vi "Main.vi"() -> ()   [LabVIEW 2013]
uses:
  <vilib>/Utility/error.llb/DialogType.ctl
  <vilib>/Utility/miscctls.llb/LVFontTypeDef.ctl
panel:
  out "Buv con ID":refnum<k5>
  out "LoadVolt":bool
  out "LoadPhase":bool
  in  "Tab Control":enum32{"ЛИНЗЫ ПОСТ. ТОКА", "ЛИНЗЫ ИМПУЛЬСНЫЕ"}(tab)
  in  "List of channels":i32(listbox)
  in  "ReadFromFile":bool
  in  "WriteToFile":bool
  out "Дата":string
  out "Время":string
  in  "Comm. current %":dbl=0.5 caption="%" min=0.0 max=100.0 step=0.5
  in  "Common curr. dec":bool
  in  "Common curr. inc":bool
  in  "ConnectAll":bool
  in  "DisconnectAll":bool
  in  "Set Output ON All":bool caption="ВЫХОДЫ ИСТОЧНИКОВ"
  out "текущий ист.":u8
  in  "SetCurrent":dbl min=0.0 max=72.0 step=0.1 format="%#.1g"
  in  "SetVoltage":dbl min=0.0 max=30.0 step=0.1 format="%#.1g"
  in  "SetCurrentB":bool
  in  "SetVoltageB":bool
  in  "SetOutputOffB":bool
  in  "SetOutputOnB":bool
  in  "ConnectChannel":bool
  in  "DisconnectChannel":bool
  in  "SetPhaseEn":bool=TRUE
  in  "BuvPhaseSetB":bool
  in  "SelectedBuvPhase":u16=7000 max=1000 step=1
  out "текущий ист. БУВ":u8
  in  "SelectedBuvOutVolt":dbl min=0.0 max=1000.0 step=0.1 format="%.1f"
  in  "SelectedBuvSetVolB":bool
  in  "Buv Table":i32(listbox)
  in  "Quit":bool=TRUE
  in  "SetCurrentAll":bool
  in  "SetVoltageAll":bool
  in  "Comm. voltage %":dbl caption="%" min=0.0 max=100.0 step=0.5
  in  "Common volt. dec":bool
  in  "Common volt. inc":bool
  in  "№":string="55"
  in  "DeleteChannel":bool
  in  "IP":string="172.16.21.19"
  in  "AddChannel":bool
  out "CURRENTSET":dbl[](array[numeric])
  in  "CurrentModulationOn":bool
  in  "Amp":dbl
  in  "CurrentModulationB":bool
  out "NAME":string[](array[string])
  out "ADRESS":string[](array[string])
  out "VIRef":refnum<vi>[](array[refnum])
  # "ВСЕ ИСТОЧНИКИ"
  # "ИСТОЧНИК №_"
  # "ИСТОЧНИК №_"
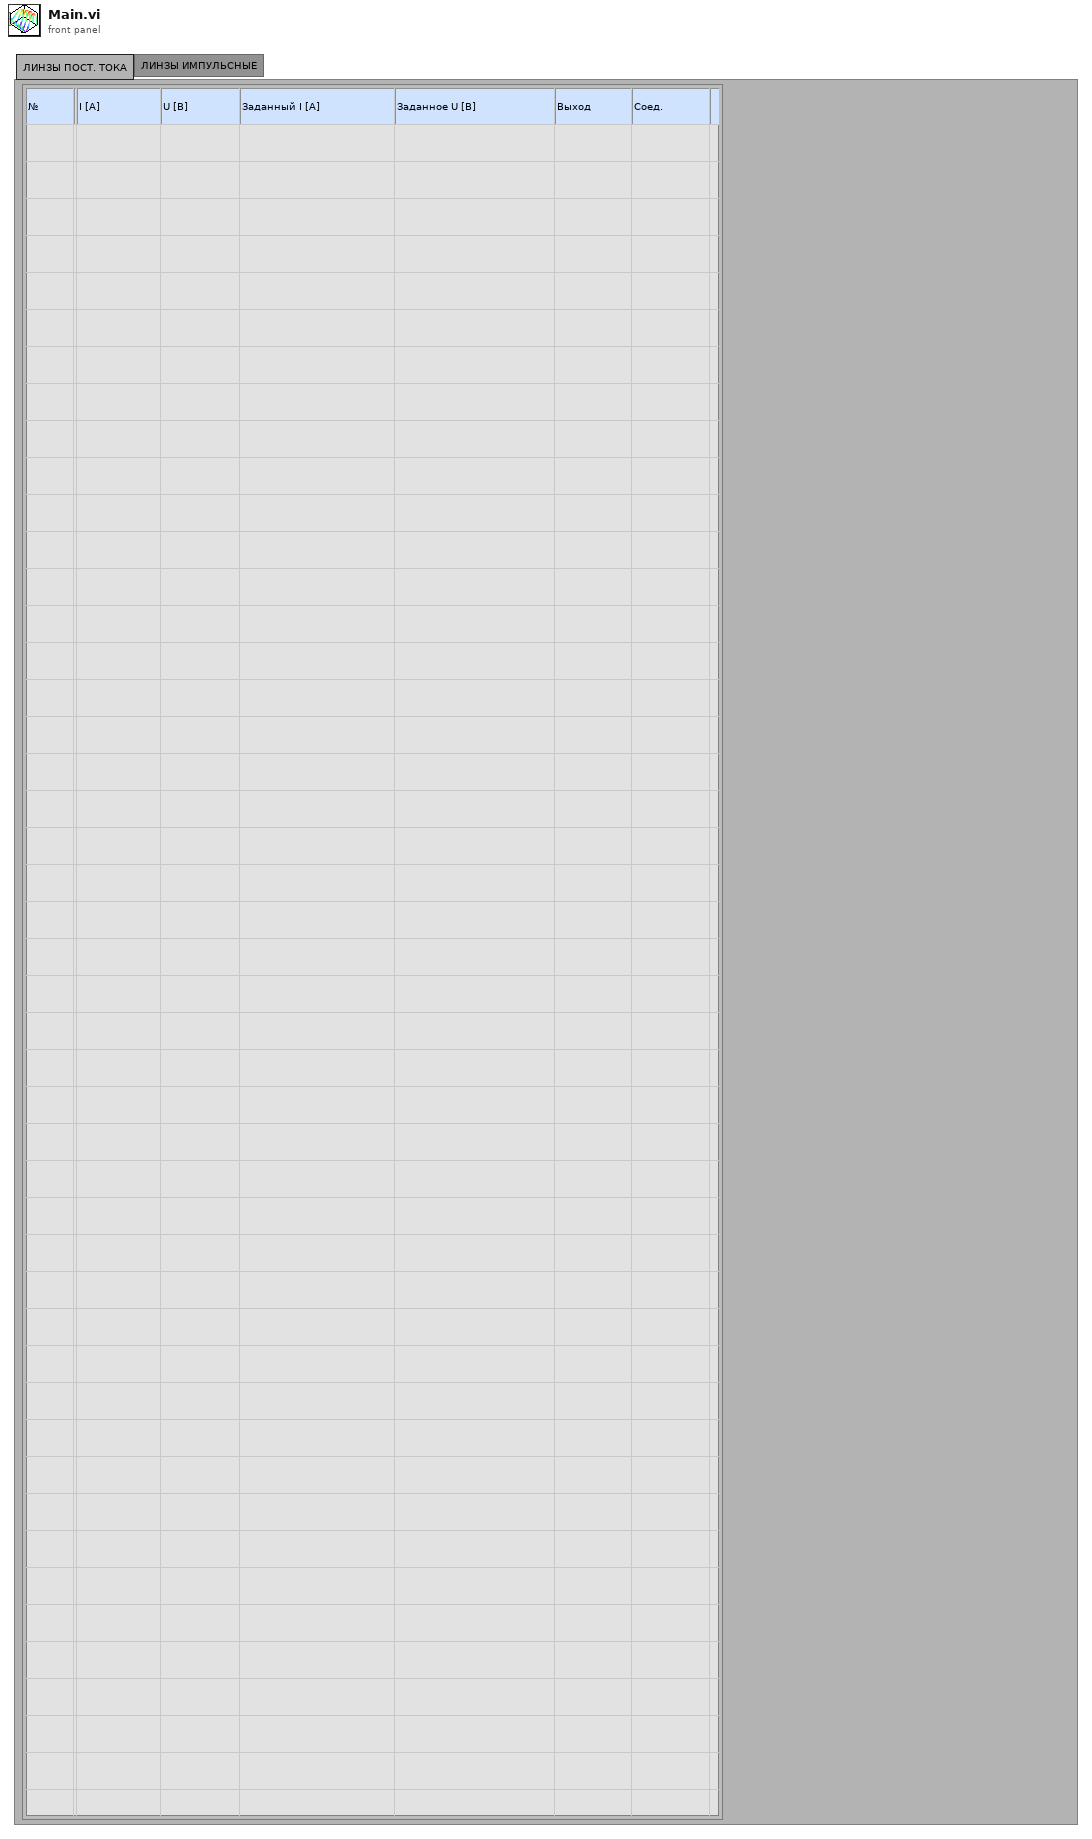
[diagram p1: front panel]
types:
  T1 = enum16{"open", "replace", "create", "open or create", "replace or create", "replace or create with confirmation"}
  T2 = enum8{"Enabled", "Disabled", "Disabled and Grayed Out"}
  T3 = typedef "DialogType.ctl" = u16
  T4 = typedef "LVFontTypeDef.ctl" = cluster{"Font Name":string, "Size":u16, "Bold":bool, "Italic":bool, "Underline":bool, "Strikeout":bool, "Color":u32}
  T5 = enum16{"Standard", "Buffered", "CRLF", "Immediate"}
  T6 = cluster{"milliseconds to wait":i32, "milliseconds to wait":i32}
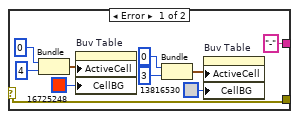
[diagram p6: hidden frame]
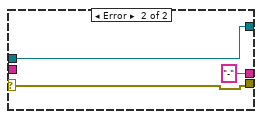
[diagram p7: hidden frame]
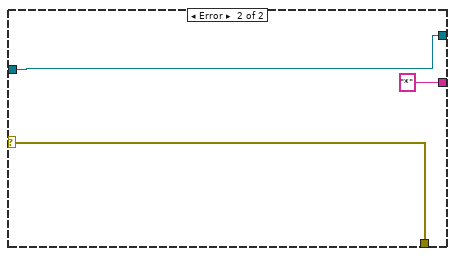
[diagram p8: hidden frame]
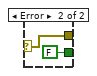
[diagram p10: hidden frame]
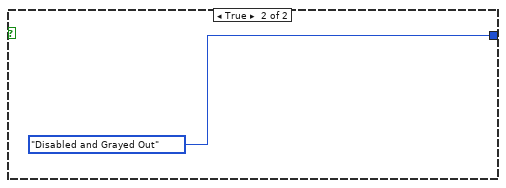
[diagram p11: hidden frame]
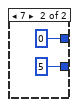
[diagram p13: hidden frame]
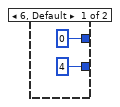
[diagram p14: hidden frame]
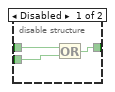
[diagram p15: hidden frame]
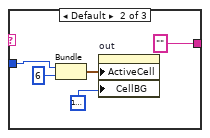
[diagram p16: hidden frame]
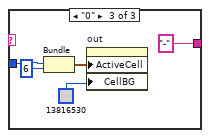
[diagram p17: hidden frame]
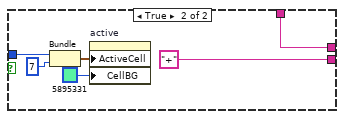
[diagram p18: hidden frame]
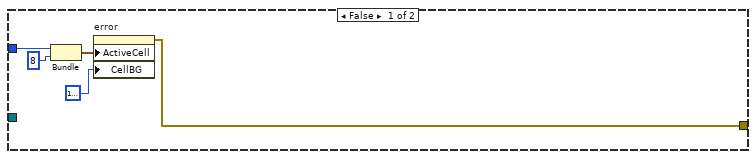
[diagram p19: hidden frame]
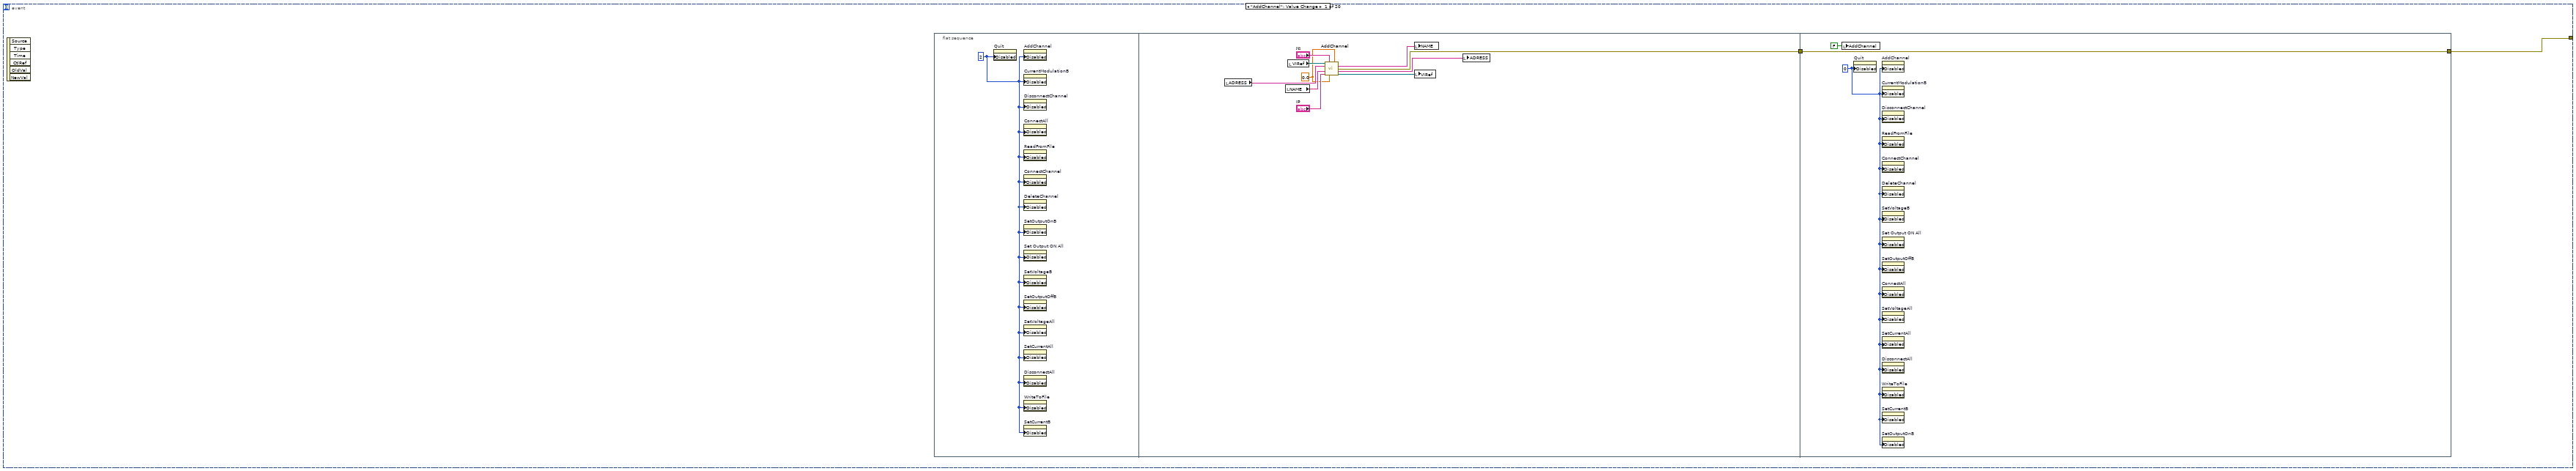
[diagram p20: hidden frame]
diagram:
  w38 = u8 0 ("Disabled")
  w40 = FALSE ("SetOutputOnB")
  w41 = FALSE ("OK Button")
  n1 = event shown="[0] \"Quit\": Value Change" {
    selector: _ -> [_]
    dyn-events: _ -> [_]
    timeout: _ -> [_]
    event "Quit": Value Change {
      n2 = event-data() -> ()  [unwired: 1 in, 1 out]
      n3 = flat-sequence {
        frame #0 {
          w46 = T3 0 items=["no dialog", "OK message", "continue or stop message", "OK message + warnings", "continue/stop + warnings"] ("type of dialog (OK msg:1)")
          n4 = local read "VIRef"() -> (w52:refnum<vi>[])
          n5 = Array Size(array=w52) -> (size(s)=w51:i32)
          n6 = for {
            N: w51 -> [_]
            tunnel: [w53] -> w49 mode=indexing
            i -> [w54]
            n7 = local read "VIRef"() -> (w57:refnum<vi>[])
            n8 = Index Array(array=w57, index=w54) -> (element=w56:refnum<vi>)
            n9 = invoke class="VI" method="Ctrl Val.Set"(reference=w56, "Control Name"="Connect", "Value"=FALSE ("OK Button")) -> (error out=w53:errorcluster)  [unwired: 2 in, 4 out]
          }
          n10 = local read "Buv con ID"() -> (w50:refnum<k5>)
          n11 = TCP Close Connection(connection ID=w50) -> (error out=w48:errorcluster)  [unwired: 2 in, 1 out]
          n12 = Merge Errors(w49, w48) -> (w47:errorcluster)
          n13 = call <vilib>:"General Error Handler.vi"("type of dialog (OK msg:1)"=w46, "error in (no error)"=w47) -> ()  [unwired: 9 in, 5 out]
        }
        frame #1 {
        }
        frame #2 {
          n14 = Stop(stop? (T)=TRUE) -> ()
        }
      }
    }
  }
  n15 = property on="Set Output ON All" class="Bool (strict)"("Disabled"=w38) -> (error out=w30:errorcluster)  [unwired: 2 in, 1 out]
  n16 = property on="SetCurrentAll" class="Bool (strict)"("Disabled"=w38) -> ()  [unwired: 2 in, 2 out]
  n17 = property on="AddChannel" class="Bool (strict)"("Disabled"=w38) -> (error out=w37:errorcluster)  [unwired: 2 in, 1 out]
  n18 = property on="AddChannel" class="Bool (strict)"("Disabled"=u8 0) -> ()  [unwired: 2 in, 2 out]
  n19 = local write "текущий ист."(u8 0 ("текущий ист.")) -> ()
  n20 = property on="IP" class="Str"("Value"="" ("IP")) -> ()  [unwired: 2 in, 2 out]
  n21 = property on="№" class="Str"("Value"="" ("Name")) -> ()  [unwired: 2 in, 2 out]
  n22 = local write "WriteToFile"(w41) -> ()
  n23 = local write "DisconnectChannel"(w41) -> ()
  n24 = local write "ConnectChannel"(w41) -> ()
  n25 = local write "SetCurrentB"(w41) -> ()
  n26 = local write "ReadFromFile"(w41) -> ()
  n27 = local write "AddChannel"(w41) -> ()
  n28 = local write "Quit"(w41) -> ()
  n29 = local write "SetCurrentAll"(w41) -> ()
  n30 = local write "SetVoltageAll"(w41) -> ()
  n31 = local write "DeleteChannel"(w41) -> ()
  n32 = local write "SetVoltageB"(w41) -> ()
  n33 = local write "SetOutputOnB"(w40) -> ()
  n34 = local write "ConnectAll"(w40) -> ()
  n35 = local write "SetOutputOffB"(w40) -> ()
  n36 = local write "DisconnectAll"(w40) -> ()
  n37 = local write "CurrentModulationB"(w40) -> ()
  n38 = local write "CurrentModulationOn"(w40) -> ()
  n39 = for "инициализация цветов и размера ячеек табл." {
    N: 50 -> [_]
    i -> [w62]
    n40 = flat-sequence {
      tunnel: w62 -> [w67]
      tunnel: [w67] -> w61
      tunnel: w61 -> [w106]
      tunnel: [w106] -> w60
      tunnel: w60 -> [w119]
      frame #0 {
        w63 = "Application font" ("Font Name")
        n41 = Bundle(w67, 4) -> (w79:cluster{i32, i32})  [unwired: 1 in]
        n42 = property on="active" class="MCListbox (strict)"("ActiveCell"=w79, "Height"=u32 35 ("Active Cell:Cell Size:Height"), "CellFontSize"=u16 28 ("Size")) -> ()  [unwired: 2 in, 2 out]
        n43 = Bundle(w67, 6) -> (w65:cluster{i32, i32})  [unwired: 1 in]
        n44 = Bundle(w67, 5) -> (w64:cluster{i32, i32})  [unwired: 1 in]
        n45 = Bundle(w67, 0) -> (w90:cluster{i32, i32})  [unwired: 1 in]
        n46 = Bundle(w67, 2) -> (w66:cluster{i32, i32})  [unwired: 1 in]
        n47 = Bundle(w67, 3) -> (w80:cluster{i32, i32})  [unwired: 1 in]
        n48 = Bundle(w67, 1) -> (w89:cluster{i32, i32})  [unwired: 1 in]
        n49 = property on="active" class="MCListbox (strict)"("ActiveCell"=w65, "Height"=u32 35 ("Active Cell:Cell Size:Height"), "CellFontSize"=u16 28 ("Size"), "CellFontName"=w63) -> ()  [unwired: 2 in, 2 out]
        n50 = property on="active" class="MCListbox (strict)"("ActiveCell"=w64, "Height"=u32 35 ("Active Cell:Cell Size:Height"), "CellFontSize"=u16 28 ("Size"), "CellFontName"=w63) -> ()  [unwired: 2 in, 2 out]
        n51 = property on="active" class="MCListbox (strict)"("ActiveCell"=w90, "Height"=u32 35 ("Active Cell:Cell Size:Height"), "CellFontSize"=u16 28 ("Size"), "CellFontName"=w63) -> ()  [unwired: 2 in, 2 out]
        n52 = property on="active" class="MCListbox (strict)"("ActiveCell"=w66, "Height"=u32 35 ("Active Cell:Cell Size:Height"), "CellFontSize"=u16 28 ("Size"), "CellFontName"=w63) -> ()  [unwired: 2 in, 2 out]
        n53 = property on="active" class="MCListbox (strict)"("ActiveCell"=w80, "Height"=u32 35 ("Active Cell:Cell Size:Height"), "CellFontSize"=u16 28 ("Size"), "CellFontName"=w63) -> ()  [unwired: 2 in, 2 out]
        n54 = property on="active" class="MCListbox (strict)"("ActiveCell"=w89, "Height"=u32 35 ("Active Cell:Cell Size:Height"), "CellFontSize"=u16 28 ("Size"), "CellFontName"=w63) -> ()  [unwired: 2 in, 2 out]
      }
      frame #1 {
        w102 = T4 {"Font Name"="Application font", "Size"=28, "Bold"=FALSE, "Italic"=FALSE, "Underline"=FALSE, "Strikeout"=FALSE, "Color"=6908265} ("Active Cell:Cell Font")
        w97 = T4 {"Font Name"="Application font", "Size"=30, "Bold"=TRUE, "Italic"=FALSE, "Underline"=FALSE, "Strikeout"=FALSE, "Color"=2263842} ("Active Cell:Cell Font")
        n55 = Bundle(w106, 4) -> (w99:cluster{i32, i32})  [unwired: 1 in]
        n56 = Bundle(w106, 3) -> (w93:cluster{i32, i32})  [unwired: 1 in]
        n57 = Bundle(w106, 2) -> (w96:cluster{i32, i32})  [unwired: 1 in]
        n58 = Bundle(w106, 0) -> (w104:cluster{i32, i32})  [unwired: 1 in]
        n59 = Bundle(w106, 5) -> (w100:cluster{i32, i32})  [unwired: 1 in]
        n60 = property on="active" class="MCListbox (strict)"("ActiveCell"=w99, "CellFont"=w102) -> ()  [unwired: 2 in, 2 out]
        n61 = property on="active" class="MCListbox (strict)"("ActiveCell"=w93, "CellFont"=w97) -> ()  [unwired: 2 in, 2 out]
        n62 = property on="active" class="MCListbox (strict)"("ActiveCell"=w96, "CellFont"=w97) -> ()  [unwired: 2 in, 2 out]
        n63 = property on="active" class="MCListbox (strict)"("ActiveCell"=w104, "CellFont"=T4 {"Font Name"="Application font", "Size"=28, "Bold"=FALSE, "Italic"=FALSE, "Underline"=FALSE, "Strikeout"=FALSE, "Color"=0} ("Active Cell:Cell Font")) -> ()  [unwired: 2 in, 2 out]
        n64 = property on="active" class="MCListbox (strict)"("ActiveCell"=w100, "CellFont"=w102) -> ()  [unwired: 2 in, 2 out]
      }
      frame #2 {
        w118 = T4 {"Font Name"="Application font", "Size"=28, "Bold"=FALSE, "Italic"=FALSE, "Underline"=FALSE, "Strikeout"=FALSE, "Color"=0} ("Active Cell:Cell Font")
        n65 = Bundle(w119, 6) -> (w113:cluster{i32, i32})  [unwired: 1 in]
        n66 = Bundle(w119, 8) -> (w114:cluster{i32, i32})  [unwired: 1 in]
        n67 = Bundle(w119, 7) -> (w115:cluster{i32, i32})  [unwired: 1 in]
        n68 = property on="active" class="MCListbox (strict)"("ActiveCell"=w113, "CellBG"=u32 16777225) -> (error out=w112:errorcluster)  [unwired: 2 in, 1 out]
        n69 = property on="error" class="MCListbox (strict)"("ActiveCell"=w114, "CellBG"=u32 16777225) -> ()  [unwired: 2 in, 2 out]
        n70 = property on="out" class="MCListbox (strict)"("ActiveCell"=w115, "CellBG"=u32 16777225) -> (error out=w116:errorcluster)  [unwired: 2 in, 1 out]
        n71 = property on="active" class="MCListbox (strict)"(error in=w112, "ActiveCell"=w113, "CellFont"=w118) -> ()  [unwired: 1 in, 2 out]
        n72 = property on="active" class="MCListbox (strict)"(error in=w116, "ActiveCell"=w115, "CellFont"=w118) -> ()  [unwired: 1 in, 2 out]
      }
    }
  }
  n73 = while {
    stop <- FALSE stop-if-true
    n74 = event shown="[13] \"SetOutputOnB\": Value Change" {
      selector: _ -> [_ _ _ _ _ _ _ _ _ _ _ _ _ _ _ _ _ _ _ _]
      dyn-events: _ -> [_ _ _ _ _ _ _ _ _ _ _ _ _ _ _ _ _ _ _ _]
      timeout: _ -> [_ _ _ _ _ _ _ _ _ _ _ _ _ _ _ _ _ _ _ _]
      tunnel: [w123 _ _ _ w227 w243 w259 w303 w347 w362 w388 w404 w420 w437 w458 w481 w499 w550 w624 w647] -> w120
      event "AddChannel": Value Change {
        n75 = event-data() -> ()  [unwired: 7 out]
        n76 = flat-sequence {
          tunnel: [w126] -> w124
          tunnel: [w136] -> w123
          tunnel: w124 -> [w136]
          frame #0 {
            w125 = u8 2 ("Disabled")
            n77 = property on="Quit" class="Bool (strict)"("Disabled"=w125) -> ()  [unwired: 2 in, 2 out]
            n78 = property on="AddChannel" class="Bool (strict)"("Disabled"=w125) -> ()  [unwired: 2 in, 2 out]
            n79 = property on="CurrentModulationB" class="Bool (strict)"("Disabled"=w125) -> ()  [unwired: 2 in, 2 out]
            n80 = property on="DisconnectChannel" class="Bool (strict)"("Disabled"=w125) -> ()  [unwired: 2 in, 2 out]
            n81 = property on="ConnectAll" class="Bool (strict)"("Disabled"=w125) -> ()  [unwired: 2 in, 2 out]
            n82 = property on="ReadFromFile" class="Bool (strict)"("Disabled"=w125) -> ()  [unwired: 2 in, 2 out]
            n83 = property on="ConnectChannel" class="Bool (strict)"("Disabled"=w125) -> ()  [unwired: 2 in, 2 out]
            n84 = property on="DeleteChannel" class="Bool (strict)"("Disabled"=w125) -> ()  [unwired: 2 in, 2 out]
            n85 = property on="SetOutputOnB" class="Bool (strict)"("Disabled"=w125) -> ()  [unwired: 2 in, 2 out]
            n86 = property on="Set Output ON All" class="Bool (strict)"("Disabled"=w125) -> ()  [unwired: 2 in, 2 out]
            n87 = property on="SetVoltageB" class="Bool (strict)"("Disabled"=w125) -> ()  [unwired: 2 in, 2 out]
            n88 = property on="SetOutputOffB" class="Bool (strict)"("Disabled"=w125) -> ()  [unwired: 2 in, 2 out]
            n89 = property on="SetVoltageAll" class="Bool (strict)"("Disabled"=w125) -> ()  [unwired: 2 in, 2 out]
            n90 = property on="SetCurrentAll" class="Bool (strict)"("Disabled"=w125) -> ()  [unwired: 2 in, 2 out]
            n91 = property on="DisconnectAll" class="Bool (strict)"("Disabled"=w125) -> ()  [unwired: 2 in, 2 out]
            n92 = property on="WriteToFile" class="Bool (strict)"("Disabled"=w125) -> ()  [unwired: 2 in, 2 out]
            n93 = property on="SetCurrentB" class="Bool (strict)"("Disabled"=w125) -> ()  [unwired: 2 in, 2 out]
          }
          frame #1 {
            w127 = 0.0 ("SetVoltage")
            n94 = local read "ADRESS"() -> (w133:string[])
            n95 = local read "NAME"() -> (w132:string[])
            n96 = local read "VIRef"() -> (w131:refnum<vi>[])
            n97 = call "AddChannel.vi"("VIRef"=w131, "Name"="№", "SetCurrent"=w127, "ADRESS"=w133, "NAME"=w132, "Address"="IP", "SetVoltage"=w127) -> ("NAMEOut"=w128:string[], "error out"=w126:errorcluster, "ADRESSOut"=w129:string[], "VIRefOut"=w130:refnum<vi>[])  [unwired: 1 in, 4 out]
            n98 = local write "NAME"(w128) -> ()
            n99 = local write "VIRef"(w130) -> ()
            n100 = local write "ADRESS"(w129) -> ()
          }
          frame #2 {
            w137 = u8 0 ("Disabled")
            n101 = local write "AddChannel"(FALSE ("AddChannel")) -> ()
            n102 = property on="Quit" class="Bool (strict)"("Disabled"=w137) -> ()  [unwired: 2 in, 2 out]
            n103 = property on="AddChannel" class="Bool (strict)"("Disabled"=w137) -> ()  [unwired: 2 in, 2 out]
            n104 = property on="CurrentModulationB" class="Bool (strict)"("Disabled"=w137) -> ()  [unwired: 2 in, 2 out]
            n105 = property on="DisconnectChannel" class="Bool (strict)"("Disabled"=w137) -> ()  [unwired: 2 in, 2 out]
            n106 = property on="ReadFromFile" class="Bool (strict)"("Disabled"=w137) -> ()  [unwired: 2 in, 2 out]
            n107 = property on="ConnectChannel" class="Bool (strict)"("Disabled"=w137) -> ()  [unwired: 2 in, 2 out]
            n108 = property on="DeleteChannel" class="Bool (strict)"("Disabled"=w137) -> ()  [unwired: 2 in, 2 out]
            n109 = property on="SetVoltageB" class="Bool (strict)"("Disabled"=w137) -> ()  [unwired: 2 in, 2 out]
            n110 = property on="Set Output ON All" class="Bool (strict)"("Disabled"=w137) -> ()  [unwired: 2 in, 2 out]
            n111 = property on="SetOutputOffB" class="Bool (strict)"("Disabled"=w137) -> ()  [unwired: 2 in, 2 out]
            n112 = property on="ConnectAll" class="Bool (strict)"("Disabled"=w137) -> ()  [unwired: 2 in, 2 out]
            n113 = property on="SetVoltageAll" class="Bool (strict)"("Disabled"=w137) -> ()  [unwired: 2 in, 2 out]
            n114 = property on="SetCurrentAll" class="Bool (strict)"("Disabled"=w137) -> ()  [unwired: 2 in, 2 out]
            n115 = property on="DisconnectAll" class="Bool (strict)"("Disabled"=w137) -> ()  [unwired: 2 in, 2 out]
            n116 = property on="WriteToFile" class="Bool (strict)"("Disabled"=w137) -> ()  [unwired: 2 in, 2 out]
            n117 = property on="SetCurrentB" class="Bool (strict)"("Disabled"=w137) -> ()  [unwired: 2 in, 2 out]
            n118 = property on="SetOutputOnB" class="Bool (strict)"("Disabled"=w137) -> ()  [unwired: 2 in, 2 out]
          }
        }
      }
      event "List of channels": Mouse Down {
        # "Работа с выбранным источником"
        n119 = event-data() -> ()  [unwired: 2 out]
        n120 = property on="List of channels" class="MCListbox (strict)"() -> ("ItemNames"=w142:string[][])  [unwired: 2 in, 2 out]
        n121 = property on="List of channels" class="MCListbox (strict)"() -> ("Value"=w141:i32)  [unwired: 2 in, 2 out]
        n122 = Index Array(array=w142, index (row)=w141) -> (element=w140:string[])  [unwired: 1 in]
        n123 = Empty Array?(array=w140) -> (empty?=w139:bool)
        n124 = case shown="False" w139 {
          tunnel: w140 -> [w143 _]
          frame False {
            n125 = flat-sequence {
              tunnel: w143 -> [w149]
              tunnel: [w149] -> w144
              tunnel: w144 -> [w162]
              frame #0 {
                n126 = Index Array(array=w149, index=0) -> (element=w152:string)
                n127 = Index Array(array=w149, index=7) -> (element=w150:string)
                n128 = case shown="\"-\", Default" w150 {
                  tunnel: [T2."Enabled" ("Disabled") T2."Disabled and Grayed Out" ("Disabled")] -> w145
                  tunnel: [w156 w158] -> w146
                  tunnel: [w156 w158] -> w148
                  tunnel: [w156 w158] -> w147
                  frame "-", Default {
                    w156 = T2."Disabled and Grayed Out" ("Disabled")
                  }
                  frame "+" {
                    w158 = T2."Enabled" ("Disabled")
                    # "соединение с ист."
                  }
                }
                n129 = Scan From String(format string="%f", input string=w152) -> (output 1=→"текущий ист.":u8)  [unwired: 3 in, 3 out]
                n130 = property on="DisconnectAll" class="Bool (strict)"("DisabledEnum"=w146) -> ()  [unwired: 2 in, 2 out]
                n131 = property on="DisconnectChannel" class="Bool (strict)"("DisabledEnum"=w146) -> ()  [unwired: 2 in, 2 out]
                n132 = property on="SetOutputOffB" class="Bool (strict)"("DisabledEnum"=w148) -> ()  [unwired: 2 in, 2 out]
                n133 = property on="SetOutputOnB" class="Bool (strict)"("DisabledEnum"=w147) -> ()  [unwired: 2 in, 2 out]
                n134 = property on="ConnectChannel" class="Bool (strict)"("DisabledEnum"=w145) -> ()  [unwired: 2 in, 2 out]
                n135 = property on="ConnectAll" class="Bool (strict)"("DisabledEnum"=w145) -> ()  [unwired: 2 in, 2 out]
              }
              frame #1 {
                n136 = Index Array(array=w162, index=5) -> (element=w167:string)
                n137 = Index Array(array=w162, index=6) -> (element=w170:string)
                n138 = Index Array(array=w162, index=4) -> (element=w164:string)
                n139 = case shown="\"+\"" w170 {
                  tunnel: [T2."Enabled" ("Disabled") T2."Disabled and Grayed Out" ("Disabled") w177] -> w171
                  tunnel: [T2."Disabled and Grayed Out" ("Disabled") T2."Enabled" ("Disabled") w177] -> w172
                  frame "-", Default {
                  }
                  frame "+" {
                  }
                  frame "?" {
                    w177 = T2."Disabled and Grayed Out" ("Disabled")
                  }
                }
                n140 = Scan From String(format string="%f", input string=w167) -> (output 1=w160:dbl)  [unwired: 3 in, 3 out]
                n141 = Scan From String(format string="%f", input string=w164) -> (output 1=w161:dbl)  [unwired: 3 in, 3 out]
                n142 = local write "SetVoltage"(w160) -> ()
                n143 = local write "SetCurrent"(w161) -> ()
                n144 = property on="SetOutputOffB" class="Bool (strict)"("DisabledEnum"=w172) -> ()  [unwired: 2 in, 2 out]
                n145 = property on="SetOutputOnB" class="Bool (strict)"("DisabledEnum"=w171) -> ()  [unwired: 2 in, 2 out]
              }
            }
          }
          frame True {
          }
        }
      }
      event "Buv Table": Mouse Down {
        # "Работа с выбранным источником БУВ"
        n146 = event-data() -> ()  [unwired: 2 out]
        n147 = property on="Buv Table" class="MCListbox (strict)"() -> ("ItemNames"=w181:string[][])  [unwired: 2 in, 2 out]
        n148 = property on="Buv Table" class="MCListbox (strict)"() -> ("Value"=w180:i32)  [unwired: 2 in, 2 out]
        n149 = Index Array(array=w181, index (row)=w180) -> (element=w179:string[])  [unwired: 1 in]
        n150 = Empty Array?(array=w179) -> (empty?=w178:bool)
        n151 = case shown="False" w178 {
          tunnel: w179 -> [w182 _]
          frame False {
            n152 = flat-sequence {
              tunnel: w182 -> [w185]
              tunnel: [w185] -> w183
              tunnel: w183 -> [w195]
              frame #0 {
                n153 = Index Array(array=w185, index=0) -> (element=w188:string)
                n154 = Index Array(array=w185, index=3) -> (element=w186:string)
                n155 = case shown="\"+\"" w186 {
                  frame "-", Default {
                  }
                  frame "+" {
                    # "соединение с ист."
                  }
                }
                n156 = Scan From String(format string="%f", input string=w188) -> (output 1=→"текущий ист. БУВ":u8)  [unwired: 3 in, 3 out]
              }
              frame #1 {
                n157 = disable-structure shown="Disabled" {
                  disable-tunnel: w195 -> [w197 _]
                  frame Disabled {
                    n158 = Index Array(array=w197, index=1) -> (element=w198:string)
                    n159 = Scan From String(format string="%f", input string=w198) -> ()  [unwired: 4 in, 3 out]
                  }
                  frame Enabled {
                  }
                }
                n160 = Index Array(array=w195, index=2) -> (element=w193:string)
                n161 = Scan From String(format string="%f", input string=w193) -> (output 1=w191:dbl)  [unwired: 3 in, 3 out]
                n162 = local write "SelectedBuvOutVolt"(w191) -> ()
              }
            }
          }
          frame True {
          }
        }
      }
      event Panel Close? {
        n163 = event-data() -> ()  [unwired: 5 out]
        n164 = Two Button Dialog(message="Вы уверены, что хотите закрыть программу?", 1:"Нет" ("F button name (\"Cancel\")"), 2:"Да" ("T button name (\"OK\")")) -> (T button?=w203:bool)
        n165 = case shown="True" w203 {
          frame False {
          }
          frame True {
            n166 = disable-structure shown="Disabled" {
              frame Disabled {
                n167 = local read item#-1() -> (w213)
                n168 = TCP Close Connection(connection ID=w213) -> ()  [unwired: 2 in, 2 out]
              }
              frame Enabled {
              }
            }
            n169 = local read "VIRef"() -> (w205:refnum<vi>[])
            n170 = Array Size(array=w205) -> (size(s)=w204:i32)
            n171 = for {
              N: w204 -> [_]
              tunnel: w205 -> [w223]
              tunnel: [w221] -> w212 mode=indexing
              i -> [w224]
              n172 = Index Array(array=w223, index=w224) -> (element=w222:refnum<vi>)
              n173 = invoke class="VI" method="Ctrl Val.Set"(reference=w222, "Control Name"="Connect", "Value"=FALSE) -> (error out=w221:errorcluster)  [unwired: 2 in, 4 out]
            }
            n174 = flat-sequence {
              tunnel: [w215] -> w211
              tunnel: w212 -> [w215]
              frame #0 {
                n175 = Wait (ms)(milliseconds to wait=u32 1000) -> ()  [unwired: 1 out]
              }
            }
            n176 = local read "VIRef"() -> (w206:refnum<vi>[])
            n177 = Array Size(array=w206) -> (size(s)=w207:i32)
            n178 = for {
              N: w207 -> [_]
              tunnel: w206 -> [w219]
              tunnel: [w217] -> w208 mode=indexing
              tunnel: w211 -> [w216] mode=indexing
              i -> [w220]
              n179 = Index Array(array=w219, index=w220) -> (element=w218:refnum<vi>)
              n180 = invoke class="VI" method="Abort VI"(reference=w218, error in=w216) -> (error out=w217:errorcluster)  [unwired: 1 in, 2 out]
            }
            n181 = Merge Errors(w208) -> (w209:errorcluster)
            n182 = call <vilib>:"General Error Handler.vi"("type of dialog (OK msg:1)"=u32 0 ("milliseconds to wait"), "error in (no error)"=w209) -> ()  [unwired: 9 in, 5 out]
          }
        }
        n183 = event-data() -> ()  [unwired: 2 in, 1 out]
      }
      event "SetVoltageAll": Value Change {
        n184 = event-data() -> ()  [unwired: 7 out]
        n185 = flat-sequence {
          tunnel: [w231] -> w229
          tunnel: [w240] -> w228
          tunnel: w229 -> [w240]
          frame #0 {
            w230 = u8 2 ("Disabled")
            n186 = property on="Quit" class="Bool (strict)"("Disabled"=w230) -> ()  [unwired: 2 in, 2 out]
            n187 = property on="AddChannel" class="Bool (strict)"("Disabled"=w230) -> ()  [unwired: 2 in, 2 out]
            n188 = property on="CurrentModulationB" class="Bool (strict)"("Disabled"=w230) -> ()  [unwired: 2 in, 2 out]
            n189 = property on="DisconnectChannel" class="Bool (strict)"("Disabled"=w230) -> ()  [unwired: 2 in, 2 out]
            n190 = property on="ConnectAll" class="Bool (strict)"("Disabled"=w230) -> ()  [unwired: 2 in, 2 out]
            n191 = property on="ReadFromFile" class="Bool (strict)"("Disabled"=w230) -> ()  [unwired: 2 in, 2 out]
            n192 = property on="ConnectChannel" class="Bool (strict)"("Disabled"=w230) -> ()  [unwired: 2 in, 2 out]
            n193 = property on="DeleteChannel" class="Bool (strict)"("Disabled"=w230) -> ()  [unwired: 2 in, 2 out]
            n194 = property on="SetVoltageB" class="Bool (strict)"("Disabled"=w230) -> ()  [unwired: 2 in, 2 out]
            n195 = property on="Set Output ON All" class="Bool (strict)"("Disabled"=w230) -> ()  [unwired: 2 in, 2 out]
            n196 = property on="SetOutputOffB" class="Bool (strict)"("Disabled"=w230) -> ()  [unwired: 2 in, 2 out]
            n197 = property on="SetVoltageAll" class="Bool (strict)"("Disabled"=w230) -> ()  [unwired: 2 in, 2 out]
            n198 = property on="SetCurrentAll" class="Bool (strict)"("Disabled"=w230) -> ()  [unwired: 2 in, 2 out]
            n199 = property on="DisconnectAll" class="Bool (strict)"("Disabled"=w230) -> ()  [unwired: 2 in, 2 out]
            n200 = property on="WriteToFile" class="Bool (strict)"("Disabled"=w230) -> ()  [unwired: 2 in, 2 out]
            n201 = property on="SetCurrentB" class="Bool (strict)"("Disabled"=w230) -> ()  [unwired: 2 in, 2 out]
            n202 = property on="SetOutputOnB" class="Bool (strict)"("Disabled"=w230) -> ()  [unwired: 2 in, 2 out]
          }
          frame #1 {
            n203 = local read "VIRef"() -> (w233:refnum<vi>[])
            n204 = Array Size(array=w233) -> (size(s)=w232:i32)
            n205 = for {
              N: w232 -> [_]
              tunnel: [w234] -> w231 mode=indexing
              i -> [w236]
              n206 = local read "VIRef"() -> (w239:refnum<vi>[])
              n207 = Index Array(array=w239, index=w236) -> (element=w235:refnum<vi>)
              n208 = invoke class="VI" method="Ctrl Val.Set"(reference=w235, "Control Name"="NeedToSetVoltage", "Value"=TRUE ("ConnectChannel")) -> (error out=w234:errorcluster)  [unwired: 2 in, 4 out]
            }
          }
          frame #2 {
            w241 = u8 0 ("Disabled")
            n209 = local write "SetVoltageAll"(FALSE ("SetVoltageAll")) -> ()
            n210 = property on="Quit" class="Bool (strict)"("Disabled"=w241) -> ()  [unwired: 2 in, 2 out]
            n211 = property on="AddChannel" class="Bool (strict)"("Disabled"=w241) -> ()  [unwired: 2 in, 2 out]
            n212 = property on="CurrentModulationB" class="Bool (strict)"("Disabled"=w241) -> ()  [unwired: 2 in, 2 out]
            n213 = property on="DisconnectChannel" class="Bool (strict)"("Disabled"=w241) -> ()  [unwired: 2 in, 2 out]
            n214 = property on="ReadFromFile" class="Bool (strict)"("Disabled"=w241) -> ()  [unwired: 2 in, 2 out]
            n215 = property on="ConnectChannel" class="Bool (strict)"("Disabled"=w241) -> ()  [unwired: 2 in, 2 out]
            n216 = property on="DeleteChannel" class="Bool (strict)"("Disabled"=w241) -> ()  [unwired: 2 in, 2 out]
            n217 = property on="WriteToFile" class="Bool (strict)"("Disabled"=w241) -> ()  [unwired: 2 in, 2 out]
            n218 = property on="Set Output ON All" class="Bool (strict)"("Disabled"=w241) -> ()  [unwired: 2 in, 2 out]
            n219 = property on="SetCurrentB" class="Bool (strict)"("Disabled"=w241) -> ()  [unwired: 2 in, 2 out]
            n220 = property on="ConnectAll" class="Bool (strict)"("Disabled"=w241) -> ()  [unwired: 2 in, 2 out]
            n221 = property on="SetOutputOnB" class="Bool (strict)"("Disabled"=w241) -> ()  [unwired: 2 in, 2 out]
            n222 = property on="SetVoltageB" class="Bool (strict)"("Disabled"=w241) -> ()  [unwired: 2 in, 2 out]
            n223 = property on="SetOutputOffB" class="Bool (strict)"("Disabled"=w241) -> ()  [unwired: 2 in, 2 out]
            n224 = property on="SetVoltageAll" class="Bool (strict)"("Disabled"=w241) -> ()  [unwired: 2 in, 2 out]
            n225 = property on="SetCurrentAll" class="Bool (strict)"("Disabled"=w241) -> ()  [unwired: 2 in, 2 out]
            n226 = property on="DisconnectAll" class="Bool (strict)"("Disabled"=w241) -> ()  [unwired: 2 in, 2 out]
          }
        }
        n227 = Merge Errors(w228) -> (w227:errorcluster)
      }
      event "SetCurrentAll": Value Change {
        n228 = event-data() -> ()  [unwired: 7 out]
        n229 = flat-sequence {
          tunnel: [w247] -> w245
          tunnel: [w256] -> w244
          tunnel: w245 -> [w256]
          frame #0 {
            w246 = u8 2 ("Disabled")
            n230 = property on="Quit" class="Bool (strict)"("Disabled"=w246) -> ()  [unwired: 2 in, 2 out]
            n231 = property on="AddChannel" class="Bool (strict)"("Disabled"=w246) -> ()  [unwired: 2 in, 2 out]
            n232 = property on="CurrentModulationB" class="Bool (strict)"("Disabled"=w246) -> ()  [unwired: 2 in, 2 out]
            n233 = property on="DisconnectChannel" class="Bool (strict)"("Disabled"=w246) -> ()  [unwired: 2 in, 2 out]
            n234 = property on="ConnectAll" class="Bool (strict)"("Disabled"=w246) -> ()  [unwired: 2 in, 2 out]
            n235 = property on="ReadFromFile" class="Bool (strict)"("Disabled"=w246) -> ()  [unwired: 2 in, 2 out]
            n236 = property on="ConnectChannel" class="Bool (strict)"("Disabled"=w246) -> ()  [unwired: 2 in, 2 out]
            n237 = property on="DeleteChannel" class="Bool (strict)"("Disabled"=w246) -> ()  [unwired: 2 in, 2 out]
            n238 = property on="SetOutputOffB" class="Bool (strict)"("Disabled"=w246) -> ()  [unwired: 2 in, 2 out]
            n239 = property on="Set Output ON All" class="Bool (strict)"("Disabled"=w246) -> ()  [unwired: 2 in, 2 out]
            n240 = property on="SetVoltageAll" class="Bool (strict)"("Disabled"=w246) -> ()  [unwired: 2 in, 2 out]
            n241 = property on="SetCurrentAll" class="Bool (strict)"("Disabled"=w246) -> ()  [unwired: 2 in, 2 out]
            n242 = property on="DisconnectAll" class="Bool (strict)"("Disabled"=w246) -> ()  [unwired: 2 in, 2 out]
            n243 = property on="WriteToFile" class="Bool (strict)"("Disabled"=w246) -> ()  [unwired: 2 in, 2 out]
            n244 = property on="SetCurrentB" class="Bool (strict)"("Disabled"=w246) -> ()  [unwired: 2 in, 2 out]
            n245 = property on="SetOutputOnB" class="Bool (strict)"("Disabled"=w246) -> ()  [unwired: 2 in, 2 out]
            n246 = property on="SetVoltageB" class="Bool (strict)"("Disabled"=w246) -> ()  [unwired: 2 in, 2 out]
          }
          frame #1 {
            n247 = local read "VIRef"() -> (w249:refnum<vi>[])
            n248 = Array Size(array=w249) -> (size(s)=w248:i32)
            n249 = for {
              N: w248 -> [_]
              tunnel: [w250] -> w247 mode=indexing
              i -> [w252]
              n250 = local read "VIRef"() -> (w255:refnum<vi>[])
              n251 = Index Array(array=w255, index=w252) -> (element=w251:refnum<vi>)
              n252 = invoke class="VI" method="Ctrl Val.Set"(reference=w251, "Control Name"="NeedToSetCurrent", "Value"=TRUE ("ConnectChannel")) -> (error out=w250:errorcluster)  [unwired: 2 in, 4 out]
            }
          }
          frame #2 {
            w257 = u8 0 ("Disabled")
            n253 = local write "SetCurrentAll"(FALSE ("SetVoltageAll")) -> ()
            n254 = property on="Quit" class="Bool (strict)"("Disabled"=w257) -> ()  [unwired: 2 in, 2 out]
            n255 = property on="AddChannel" class="Bool (strict)"("Disabled"=w257) -> ()  [unwired: 2 in, 2 out]
            n256 = property on="CurrentModulationB" class="Bool (strict)"("Disabled"=w257) -> ()  [unwired: 2 in, 2 out]
            n257 = property on="DisconnectChannel" class="Bool (strict)"("Disabled"=w257) -> ()  [unwired: 2 in, 2 out]
            n258 = property on="ReadFromFile" class="Bool (strict)"("Disabled"=w257) -> ()  [unwired: 2 in, 2 out]
            n259 = property on="ConnectChannel" class="Bool (strict)"("Disabled"=w257) -> ()  [unwired: 2 in, 2 out]
            n260 = property on="DeleteChannel" class="Bool (strict)"("Disabled"=w257) -> ()  [unwired: 2 in, 2 out]
            n261 = property on="WriteToFile" class="Bool (strict)"("Disabled"=w257) -> ()  [unwired: 2 in, 2 out]
            n262 = property on="Set Output ON All" class="Bool (strict)"("Disabled"=w257) -> ()  [unwired: 2 in, 2 out]
            n263 = property on="SetCurrentB" class="Bool (strict)"("Disabled"=w257) -> ()  [unwired: 2 in, 2 out]
            n264 = property on="ConnectAll" class="Bool (strict)"("Disabled"=w257) -> ()  [unwired: 2 in, 2 out]
            n265 = property on="SetOutputOnB" class="Bool (strict)"("Disabled"=w257) -> ()  [unwired: 2 in, 2 out]
            n266 = property on="SetVoltageB" class="Bool (strict)"("Disabled"=w257) -> ()  [unwired: 2 in, 2 out]
            n267 = property on="SetOutputOffB" class="Bool (strict)"("Disabled"=w257) -> ()  [unwired: 2 in, 2 out]
            n268 = property on="SetVoltageAll" class="Bool (strict)"("Disabled"=w257) -> ()  [unwired: 2 in, 2 out]
            n269 = property on="SetCurrentAll" class="Bool (strict)"("Disabled"=w257) -> ()  [unwired: 2 in, 2 out]
            n270 = property on="DisconnectAll" class="Bool (strict)"("Disabled"=w257) -> ()  [unwired: 2 in, 2 out]
          }
        }
        n271 = Merge Errors(w244) -> (w243:errorcluster)
      }
      event "Common curr. inc", "Common curr. dec": Value Change {
        # "Общее управление токами"
        n272 = event-data() -> ()  [unwired: 2 out]
        n273 = local read "ADRESS"() -> (w262:string[])
        n274 = Array Size(array=w262) -> (size(s)=w263:i32)
        n275 = for {
          N: w263 -> [_]
          tunnel: [w272] -> w261 mode=indexing
          i -> [w290]
          n276 = local read "VIRef"() -> (w293:refnum<vi>[])
          n277 = Index Array(array=w293, index=w290) -> (element=w280:refnum<vi>)
          n278 = invoke class="VI" method="Ctrl Val.Get"(reference=w280, "Control Name"="SetCurrentStr") -> (reference out=w274:refnum<vi>, error out=w288:errorcluster, "Get Control Value Variant"=w292:variant)  [unwired: 2 in, 1 out]
          n279 = Variant To Data(error in=w288, type="" ("Control Name"), Variant=w292) -> (data=w287:string, error out=w286:errorcluster)
          n280 = Scan From String(format string="%f", input string=w287, error in=w286) -> (error out=w273:errorcluster, output 1=w271:dbl)  [unwired: 2 in, 2 out]
          n281 = Multiply(x=w271, y="Comm. current %") -> (x*y=w282:dbl)
          n282 = Divide(x=w282, y=100.0) -> (x/y=w284:dbl)
          n283 = local read "Common curr. inc"() -> (w270:bool)
          n284 = local read "Common curr. dec"() -> (w268:bool)
          n285 = case shown="True" w270 {
            tunnel: w284 -> [w298 w302]
            tunnel: w271 -> [w299 w301]
            tunnel: [w299 w300] -> w269
            tunnel: [w298 _] -> w267
            frame False {
            }
            frame True {
              n286 = Add(x=w301, y=w302) -> (x+y=w300:dbl)
            }
          }
          n287 = case shown="False" w268 {
            tunnel: w269 -> [w294 w297]
            tunnel: [w294 w296] -> w266
            tunnel: w267 -> [_ w295]
            frame False {
            }
            frame True {
              n288 = Subtract(x=w297, y=w295) -> (x-y=w296:dbl)
            }
          }
          n289 = invoke class="VI" method="Ctrl Val.Set"(reference=w274, error in=w273, "Control Name"="SetCurrent", "Value"=w266) -> (reference out=w276:refnum<vi>, error out=w275:errorcluster)  [unwired: 1 in, 3 out]
          n290 = invoke class="VI" method="Ctrl Val.Set"(reference=w276, error in=w275, "Control Name"="NeedToSetCurrent", "Value"=TRUE ("ConnectChannel")) -> (error out=w272:errorcluster)  [unwired: 1 in, 4 out]
        }
        n291 = Merge Errors(w261) -> (w260:errorcluster)
        n292 = flat-sequence {
          tunnel: w260 -> [w265]
          tunnel: [w265] -> w259
          frame #0 {
            w264 = FALSE ("ConnectChannel")
            n293 = local write "Common curr. inc"(w264) -> ()
            n294 = local write "Common curr. dec"(w264) -> ()
          }
        }
      }
      event "Common volt. inc", "Common volt. dec": Value Change {
        # "Общее управление напряжением"
        n295 = event-data() -> ()  [unwired: 2 out]
        n296 = local read "ADRESS"() -> (w306:string[])
        n297 = Array Size(array=w306) -> (size(s)=w307:i32)
        n298 = for {
          N: w307 -> [_]
          tunnel: [w317] -> w305 mode=indexing
          i -> [w334]
          n299 = local read "VIRef"() -> (w337:refnum<vi>[])
          n300 = Index Array(array=w337, index=w334) -> (element=w325:refnum<vi>)
          n301 = invoke class="VI" method="Ctrl Val.Get"(reference=w325, "Control Name"="SetVoltageStr") -> (reference out=w319:refnum<vi>, error out=w332:errorcluster, "Get Control Value Variant"=w336:variant)  [unwired: 2 in, 1 out]
          n302 = Variant To Data(error in=w332, type="" ("Control Name"), Variant=w336) -> (data=w331:string, error out=w330:errorcluster)
          n303 = Scan From String(format string="%f", input string=w331, error in=w330) -> (error out=w318:errorcluster, output 1=w316:dbl)  [unwired: 2 in, 2 out]
          n304 = Multiply(x=w316, y="Comm. voltage %") -> (x*y=w326:dbl)
          n305 = Divide(x=w326, y=100.0) -> (x/y=w328:dbl)
          n306 = local read "Common volt. inc"() -> (w315:bool)
          n307 = local read "Common volt. dec"() -> (w313:bool)
          n308 = case shown="True" w315 {
            tunnel: w328 -> [w342 w346]
            tunnel: w316 -> [w343 w345]
            tunnel: [w343 w344] -> w314
            tunnel: [w342 _] -> w312
            frame False {
            }
            frame True {
              n309 = Add(x=w345, y=w346) -> (x+y=w344:dbl)
            }
          }
          n310 = case shown="False" w313 {
            tunnel: w314 -> [w338 w341]
            tunnel: [w338 w340] -> w311
            tunnel: w312 -> [_ w339]
            frame False {
            }
            frame True {
              n311 = Subtract(x=w341, y=w339) -> (x-y=w340:dbl)
            }
          }
          n312 = invoke class="VI" method="Ctrl Val.Set"(reference=w319, error in=w318, "Control Name"="SetVoltage", "Value"=w311) -> (reference out=w321:refnum<vi>, error out=w320:errorcluster)  [unwired: 1 in, 3 out]
          n313 = invoke class="VI" method="Ctrl Val.Set"(reference=w321, error in=w320, "Control Name"="NeedToSetVoltage", "Value"=TRUE ("ConnectChannel")) -> (error out=w317:errorcluster)  [unwired: 1 in, 4 out]
        }
        n314 = Merge Errors(w305) -> (w304:errorcluster)
        n315 = flat-sequence {
          tunnel: w304 -> [w309]
          tunnel: [w309] -> w303
          frame #0 {
            w308 = FALSE ("ConnectChannel")
            n316 = local write "Common volt. inc"(w308) -> ()
            n317 = local write "Common volt. dec"(w308) -> ()
          }
        }
      }
      event "DisconnectChannel": Value Change {
        n318 = event-data() -> ()  [unwired: 7 out]
        n319 = property on="List of channels" class="MCListbox (strict)"() -> ("Value"=w351:i32)  [unwired: 2 in, 2 out]
        n320 = flat-sequence {
          tunnel: w351 -> [w353]
          tunnel: [w353] -> w350
          tunnel: w350 -> [w355]
          tunnel: [w354] -> w348
          tunnel: [w360] -> w349
          tunnel: w348 -> [w360]
          frame #0 {
            w352 = u8 2 ("Disabled")
            n321 = property on="AddChannel" class="Bool (strict)"("Disabled"=w352) -> ()  [unwired: 2 in, 2 out]
            n322 = property on="Set Output ON All" class="Bool (strict)"("Disabled"=w352) -> ()  [unwired: 2 in, 2 out]
            n323 = property on="CurrentModulationB" class="Bool (strict)"("Disabled"=w352) -> ()  [unwired: 2 in, 2 out]
            n324 = property on="ConnectAll" class="Bool (strict)"("Disabled"=w352) -> ()  [unwired: 2 in, 2 out]
            n325 = property on="DisconnectChannel" class="Bool (strict)"("Disabled"=w352) -> ()  [unwired: 2 in, 2 out]
            n326 = property on="ReadFromFile" class="Bool (strict)"("Disabled"=w352) -> ()  [unwired: 2 in, 2 out]
            n327 = property on="Quit" class="Bool (strict)"("Disabled"=w352) -> ()  [unwired: 2 in, 2 out]
            n328 = property on="ConnectChannel" class="Bool (strict)"("Disabled"=w352) -> ()  [unwired: 2 in, 2 out]
            n329 = property on="DeleteChannel" class="Bool (strict)"("Disabled"=w352) -> ()  [unwired: 2 in, 2 out]
            n330 = property on="WriteToFile" class="Bool (strict)"("Disabled"=w352) -> ()  [unwired: 2 in, 2 out]
            n331 = property on="SetCurrentB" class="Bool (strict)"("Disabled"=w352) -> ()  [unwired: 2 in, 2 out]
            n332 = property on="SetOutputOnB" class="Bool (strict)"("Disabled"=w352) -> ()  [unwired: 2 in, 2 out]
            n333 = property on="SetVoltageB" class="Bool (strict)"("Disabled"=w352) -> ()  [unwired: 2 in, 2 out]
            n334 = property on="SetOutputOffB" class="Bool (strict)"("Disabled"=w352) -> ()  [unwired: 2 in, 2 out]
            n335 = property on="SetVoltageAll" class="Bool (strict)"("Disabled"=w352) -> ()  [unwired: 2 in, 2 out]
            n336 = property on="SetCurrentAll" class="Bool (strict)"("Disabled"=w352) -> ()  [unwired: 2 in, 2 out]
            n337 = property on="DisconnectAll" class="Bool (strict)"("Disabled"=w352) -> ()  [unwired: 2 in, 2 out]
          }
          frame #1 {
            w356 = FALSE ("OK Button")
            n338 = local write "DisconnectChannel"(w356) -> ()
            n339 = local read "VIRef"() -> (w358:refnum<vi>[])
            n340 = Index Array(array=w358, index=w355) -> (element=w357:refnum<vi>)
            n341 = invoke class="VI" method="Ctrl Val.Set"(reference=w357, "Control Name"="Connect", "Value"=w356) -> (error out=w354:errorcluster)  [unwired: 2 in, 4 out]
          }
          frame #2 {
            w361 = u8 0 ("Disabled")
            n342 = property on="AddChannel" class="Bool (strict)"("Disabled"=w361) -> ()  [unwired: 2 in, 2 out]
            n343 = property on="CurrentModulationB" class="Bool (strict)"("Disabled"=w361) -> ()  [unwired: 2 in, 2 out]
            n344 = property on="DisconnectChannel" class="Bool (strict)"("Disabled"=w361) -> ()  [unwired: 2 in, 2 out]
            n345 = property on="ConnectAll" class="Bool (strict)"("Disabled"=w361) -> ()  [unwired: 2 in, 2 out]
            n346 = property on="ReadFromFile" class="Bool (strict)"("Disabled"=w361) -> ()  [unwired: 2 in, 2 out]
            n347 = property on="ConnectChannel" class="Bool (strict)"("Disabled"=w361) -> ()  [unwired: 2 in, 2 out]
            n348 = property on="Quit" class="Bool (strict)"("Disabled"=w361) -> ()  [unwired: 2 in, 2 out]
            n349 = property on="DeleteChannel" class="Bool (strict)"("Disabled"=w361) -> ()  [unwired: 2 in, 2 out]
            n350 = property on="SetOutputOffB" class="Bool (strict)"("Disabled"=w361) -> ()  [unwired: 2 in, 2 out]
            n351 = property on="Set Output ON All" class="Bool (strict)"("Disabled"=w361) -> ()  [unwired: 2 in, 2 out]
            n352 = property on="SetVoltageAll" class="Bool (strict)"("Disabled"=w361) -> ()  [unwired: 2 in, 2 out]
            n353 = property on="SetCurrentAll" class="Bool (strict)"("Disabled"=w361) -> ()  [unwired: 2 in, 2 out]
            n354 = property on="DisconnectAll" class="Bool (strict)"("Disabled"=w361) -> ()  [unwired: 2 in, 2 out]
            n355 = property on="WriteToFile" class="Bool (strict)"("Disabled"=w361) -> ()  [unwired: 2 in, 2 out]
            n356 = property on="SetCurrentB" class="Bool (strict)"("Disabled"=w361) -> ()  [unwired: 2 in, 2 out]
            n357 = property on="SetOutputOnB" class="Bool (strict)"("Disabled"=w361) -> ()  [unwired: 2 in, 2 out]
            n358 = property on="SetVoltageB" class="Bool (strict)"("Disabled"=w361) -> ()  [unwired: 2 in, 2 out]
          }
        }
        n359 = Merge Errors(w349) -> (w347:errorcluster)
      }
      event "ConnectChannel": Value Change {
        n360 = event-data() -> ()  [unwired: 7 out]
        n361 = property on="List of channels" class="MCListbox (strict)"() -> ("Value"=w366:i32)  [unwired: 2 in, 2 out]
        n362 = flat-sequence {
          tunnel: w366 -> [w368]
          tunnel: [w368] -> w365
          tunnel: w365 -> [w373]
          tunnel: [w372] -> w363
          tunnel: [w385] -> w364
          tunnel: w363 -> [w385]
          frame #0 {
            w367 = u8 2 ("Disabled")
            n363 = property on="AddChannel" class="Bool (strict)"("Disabled"=w367) -> ()  [unwired: 2 in, 2 out]
            n364 = property on="Set Output ON All" class="Bool (strict)"("Disabled"=w367) -> ()  [unwired: 2 in, 2 out]
            n365 = property on="CurrentModulationB" class="Bool (strict)"("Disabled"=w367) -> ()  [unwired: 2 in, 2 out]
            n366 = property on="ConnectAll" class="Bool (strict)"("Disabled"=w367) -> ()  [unwired: 2 in, 2 out]
            n367 = property on="DisconnectChannel" class="Bool (strict)"("Disabled"=w367) -> ()  [unwired: 2 in, 2 out]
            n368 = property on="ReadFromFile" class="Bool (strict)"("Disabled"=w367) -> ()  [unwired: 2 in, 2 out]
            n369 = property on="Quit" class="Bool (strict)"("Disabled"=w367) -> ()  [unwired: 2 in, 2 out]
            n370 = property on="ConnectChannel" class="Bool (strict)"("Disabled"=w367) -> ()  [unwired: 2 in, 2 out]
            n371 = property on="DeleteChannel" class="Bool (strict)"("Disabled"=w367) -> ()  [unwired: 2 in, 2 out]
            n372 = property on="WriteToFile" class="Bool (strict)"("Disabled"=w367) -> ()  [unwired: 2 in, 2 out]
            n373 = property on="SetCurrentB" class="Bool (strict)"("Disabled"=w367) -> ()  [unwired: 2 in, 2 out]
            n374 = property on="SetOutputOnB" class="Bool (strict)"("Disabled"=w367) -> ()  [unwired: 2 in, 2 out]
            n375 = property on="SetVoltageB" class="Bool (strict)"("Disabled"=w367) -> ()  [unwired: 2 in, 2 out]
            n376 = property on="SetOutputOffB" class="Bool (strict)"("Disabled"=w367) -> ()  [unwired: 2 in, 2 out]
            n377 = property on="SetVoltageAll" class="Bool (strict)"("Disabled"=w367) -> ()  [unwired: 2 in, 2 out]
            n378 = property on="SetCurrentAll" class="Bool (strict)"("Disabled"=w367) -> ()  [unwired: 2 in, 2 out]
            n379 = property on="DisconnectAll" class="Bool (strict)"("Disabled"=w367) -> ()  [unwired: 2 in, 2 out]
          }
          frame #1 {
            n380 = local read "VIRef"() -> (w374:refnum<vi>[])
            n381 = Index Array(array=w374, index=w373) -> (element=w371:refnum<vi>)
            n382 = flat-sequence {
              tunnel: w371 -> [w376]
              tunnel: [w375] -> w369
              tunnel: [w379] -> w370
              tunnel: w369 -> [w379]
              tunnel: [w381] -> w372
              tunnel: w370 -> [w382]
              frame #0 {
                n383 = invoke class="VI" method="Ctrl Val.Set"(reference=w376, "Control Name"="Connect", "Value"=FALSE ("OK Button")) -> (reference out=w375:refnum<vi>)  [unwired: 2 in, 4 out]
              }
              frame #1 {
                n384 = Wait (ms)(milliseconds to wait=u32 1000) -> ()  [unwired: 1 out]
              }
              frame #2 {
                n385 = invoke class="VI" method="Ctrl Val.Set"(reference=w382, "Control Name"="Connect", "Value"=TRUE ("OK Button")) -> (error out=w381:errorcluster)  [unwired: 2 in, 4 out]
              }
            }
          }
          frame #2 {
            w386 = u8 0 ("Disabled")
            n386 = local write "ConnectChannel"(FALSE ("ConnectChannel")) -> ()
            n387 = property on="ConnectAll" class="Bool (strict)"("Disabled"=w386) -> ()  [unwired: 2 in, 2 out]
            n388 = property on="Set Output ON All" class="Bool (strict)"("Disabled"=w386) -> ()  [unwired: 2 in, 2 out]
            n389 = property on="AddChannel" class="Bool (strict)"("Disabled"=w386) -> ()  [unwired: 2 in, 2 out]
            n390 = property on="DisconnectChannel" class="Bool (strict)"("Disabled"=w386) -> ()  [unwired: 2 in, 2 out]
            n391 = property on="ReadFromFile" class="Bool (strict)"("Disabled"=w386) -> ()  [unwired: 2 in, 2 out]
            n392 = property on="ConnectChannel" class="Bool (strict)"("Disabled"=w386) -> ()  [unwired: 2 in, 2 out]
            n393 = property on="Quit" class="Bool (strict)"("Disabled"=w386) -> ()  [unwired: 2 in, 2 out]
            n394 = property on="DeleteChannel" class="Bool (strict)"("Disabled"=w386) -> ()  [unwired: 2 in, 2 out]
            n395 = property on="WriteToFile" class="Bool (strict)"("Disabled"=w386) -> ()  [unwired: 2 in, 2 out]
            n396 = property on="CurrentModulationB" class="Bool (strict)"("Disabled"=w386) -> ()  [unwired: 2 in, 2 out]
            n397 = property on="SetCurrentB" class="Bool (strict)"("Disabled"=w386) -> ()  [unwired: 2 in, 2 out]
            n398 = property on="SetOutputOnB" class="Bool (strict)"("Disabled"=w386) -> ()  [unwired: 2 in, 2 out]
            n399 = property on="SetVoltageB" class="Bool (strict)"("Disabled"=w386) -> ()  [unwired: 2 in, 2 out]
            n400 = property on="SetOutputOffB" class="Bool (strict)"("Disabled"=w386) -> ()  [unwired: 2 in, 2 out]
            n401 = property on="SetVoltageAll" class="Bool (strict)"("Disabled"=w386) -> ()  [unwired: 2 in, 2 out]
            n402 = property on="SetCurrentAll" class="Bool (strict)"("Disabled"=w386) -> ()  [unwired: 2 in, 2 out]
            n403 = property on="DisconnectAll" class="Bool (strict)"("Disabled"=w386) -> ()  [unwired: 2 in, 2 out]
          }
        }
        n404 = Merge Errors(w364) -> (w362:errorcluster)
      }
      event "ConnectAll": Value Change {
        n405 = event-data() -> ()  [unwired: 7 out]
        n406 = flat-sequence {
          tunnel: [w392] -> w389
          tunnel: [w401] -> w390
          tunnel: w389 -> [w401]
          frame #0 {
            w391 = u8 2 ("Disabled")
            n407 = property on="Quit" class="Bool (strict)"("Disabled"=w391) -> ()  [unwired: 2 in, 2 out]
            n408 = property on="ReadFromFile" class="Bool (strict)"("Disabled"=w391) -> ()  [unwired: 2 in, 2 out]
            n409 = property on="CurrentModulationB" class="Bool (strict)"("Disabled"=w391) -> ()  [unwired: 2 in, 2 out]
            n410 = property on="WriteToFile" class="Bool (strict)"("Disabled"=w391) -> ()  [unwired: 2 in, 2 out]
            n411 = property on="ConnectAll" class="Bool (strict)"("Disabled"=w391) -> ()  [unwired: 2 in, 2 out]
            n412 = property on="Set Output ON All" class="Bool (strict)"("Disabled"=w391) -> ()  [unwired: 2 in, 2 out]
            n413 = property on="SetOutputOffB" class="Bool (strict)"("Disabled"=w391) -> ()  [unwired: 2 in, 2 out]
            n414 = property on="AddChannel" class="Bool (strict)"("Disabled"=w391) -> ()  [unwired: 2 in, 2 out]
            n415 = property on="DisconnectChannel" class="Bool (strict)"("Disabled"=w391) -> ()  [unwired: 2 in, 2 out]
            n416 = property on="SetCurrentAll" class="Bool (strict)"("Disabled"=w391) -> ()  [unwired: 2 in, 2 out]
            n417 = property on="SetOutputOnB" class="Bool (strict)"("Disabled"=w391) -> ()  [unwired: 2 in, 2 out]
            n418 = property on="ConnectChannel" class="Bool (strict)"("Disabled"=w391) -> ()  [unwired: 2 in, 2 out]
            n419 = property on="DeleteChannel" class="Bool (strict)"("Disabled"=w391) -> ()  [unwired: 2 in, 2 out]
            n420 = property on="SetCurrentB" class="Bool (strict)"("Disabled"=w391) -> ()  [unwired: 2 in, 2 out]
            n421 = property on="SetVoltageB" class="Bool (strict)"("Disabled"=w391) -> ()  [unwired: 2 in, 2 out]
            n422 = property on="SetVoltageAll" class="Bool (strict)"("Disabled"=w391) -> ()  [unwired: 2 in, 2 out]
            n423 = property on="DisconnectAll" class="Bool (strict)"("Disabled"=w391) -> ()  [unwired: 2 in, 2 out]
          }
          frame #1 {
            n424 = local read "VIRef"() -> (w394:refnum<vi>[])
            n425 = Array Size(array=w394) -> (size(s)=w393:i32)
            n426 = for {
              N: w393 -> [_]
              tunnel: [w395] -> w392 mode=indexing
              i -> [w396]
              n427 = local read "VIRef"() -> (w399:refnum<vi>[])
              n428 = Index Array(array=w399, index=w396) -> (element=w398:refnum<vi>)
              n429 = invoke class="VI" method="Ctrl Val.Set"(reference=w398, "Control Name"="Connect", "Value"=TRUE ("OK Button")) -> (error out=w395:errorcluster)  [unwired: 2 in, 4 out]
            }
          }
          frame #2 {
            w402 = u8 0 ("Disabled")
            n430 = local write "ConnectAll"(FALSE ("ConnectChannel")) -> ()
            n431 = property on="Quit" class="Bool (strict)"("Disabled"=w402) -> ()  [unwired: 2 in, 2 out]
            n432 = property on="AddChannel" class="Bool (strict)"("Disabled"=w402) -> ()  [unwired: 2 in, 2 out]
            n433 = property on="DisconnectChannel" class="Bool (strict)"("Disabled"=w402) -> ()  [unwired: 2 in, 2 out]
            n434 = property on="ConnectAll" class="Bool (strict)"("Disabled"=w402) -> ()  [unwired: 2 in, 2 out]
            n435 = property on="Set Output ON All" class="Bool (strict)"("Disabled"=w402) -> ()  [unwired: 2 in, 2 out]
            n436 = property on="SetOutputOffB" class="Bool (strict)"("Disabled"=w402) -> ()  [unwired: 2 in, 2 out]
            n437 = property on="SetCurrentAll" class="Bool (strict)"("Disabled"=w402) -> ()  [unwired: 2 in, 2 out]
            n438 = property on="ConnectChannel" class="Bool (strict)"("Disabled"=w402) -> ()  [unwired: 2 in, 2 out]
            n439 = property on="SetVoltageAll" class="Bool (strict)"("Disabled"=w402) -> ()  [unwired: 2 in, 2 out]
            n440 = property on="SetOutputOnB" class="Bool (strict)"("Disabled"=w402) -> ()  [unwired: 2 in, 2 out]
            n441 = property on="CurrentModulationB" class="Bool (strict)"("Disabled"=w402) -> ()  [unwired: 2 in, 2 out]
            n442 = property on="DisconnectAll" class="Bool (strict)"("Disabled"=w402) -> ()  [unwired: 2 in, 2 out]
            n443 = property on="ReadFromFile" class="Bool (strict)"("Disabled"=w402) -> ()  [unwired: 2 in, 2 out]
            n444 = property on="WriteToFile" class="Bool (strict)"("Disabled"=w402) -> ()  [unwired: 2 in, 2 out]
            n445 = property on="SetCurrentB" class="Bool (strict)"("Disabled"=w402) -> ()  [unwired: 2 in, 2 out]
            n446 = property on="SetVoltageB" class="Bool (strict)"("Disabled"=w402) -> ()  [unwired: 2 in, 2 out]
            n447 = property on="DeleteChannel" class="Bool (strict)"("Disabled"=w402) -> ()  [unwired: 2 in, 2 out]
          }
        }
        n448 = Merge Errors(w390) -> (w388:errorcluster)
      }
      event "DisconnectAll": Value Change {
        n449 = event-data() -> ()  [unwired: 7 out]
        n450 = flat-sequence {
          tunnel: [w408] -> w406
          tunnel: [w417] -> w405
          tunnel: w406 -> [w417]
          frame #0 {
            w407 = u8 2 ("Disabled")
            n451 = property on="Quit" class="Bool (strict)"("Disabled"=w407) -> ()  [unwired: 2 in, 2 out]
            n452 = property on="ReadFromFile" class="Bool (strict)"("Disabled"=w407) -> ()  [unwired: 2 in, 2 out]
            n453 = property on="CurrentModulationB" class="Bool (strict)"("Disabled"=w407) -> ()  [unwired: 2 in, 2 out]
            n454 = property on="ConnectAll" class="Bool (strict)"("Disabled"=w407) -> ()  [unwired: 2 in, 2 out]
            n455 = property on="ConnectChannel" class="Bool (strict)"("Disabled"=w407) -> ()  [unwired: 2 in, 2 out]
            n456 = property on="AddChannel" class="Bool (strict)"("Disabled"=w407) -> ()  [unwired: 2 in, 2 out]
            n457 = property on="DisconnectChannel" class="Bool (strict)"("Disabled"=w407) -> ()  [unwired: 2 in, 2 out]
            n458 = property on="Set Output ON All" class="Bool (strict)"("Disabled"=w407) -> ()  [unwired: 2 in, 2 out]
            n459 = property on="WriteToFile" class="Bool (strict)"("Disabled"=w407) -> ()  [unwired: 2 in, 2 out]
            n460 = property on="SetOutputOffB" class="Bool (strict)"("Disabled"=w407) -> ()  [unwired: 2 in, 2 out]
            n461 = property on="SetCurrentAll" class="Bool (strict)"("Disabled"=w407) -> ()  [unwired: 2 in, 2 out]
            n462 = property on="SetOutputOnB" class="Bool (strict)"("Disabled"=w407) -> ()  [unwired: 2 in, 2 out]
            n463 = property on="DeleteChannel" class="Bool (strict)"("Disabled"=w407) -> ()  [unwired: 2 in, 2 out]
            n464 = property on="SetCurrentB" class="Bool (strict)"("Disabled"=w407) -> ()  [unwired: 2 in, 2 out]
            n465 = property on="SetVoltageB" class="Bool (strict)"("Disabled"=w407) -> ()  [unwired: 2 in, 2 out]
            n466 = property on="SetVoltageAll" class="Bool (strict)"("Disabled"=w407) -> ()  [unwired: 2 in, 2 out]
            n467 = property on="DisconnectAll" class="Bool (strict)"("Disabled"=w407) -> ()  [unwired: 2 in, 2 out]
          }
          frame #1 {
            n468 = local read "VIRef"() -> (w410:refnum<vi>[])
            n469 = Array Size(array=w410) -> (size(s)=w409:i32)
            n470 = for {
              N: w409 -> [_]
              tunnel: [w411] -> w408 mode=indexing
              i -> [w412]
              n471 = local read "VIRef"() -> (w415:refnum<vi>[])
              n472 = Index Array(array=w415, index=w412) -> (element=w414:refnum<vi>)
              n473 = invoke class="VI" method="Ctrl Val.Set"(reference=w414, "Control Name"="Connect", "Value"=FALSE ("OK Button")) -> (error out=w411:errorcluster)  [unwired: 2 in, 4 out]
            }
          }
          frame #2 {
            w418 = u8 0 ("Disabled")
            n474 = local write "DisconnectAll"(FALSE ("ConnectChannel")) -> ()
            n475 = property on="Quit" class="Bool (strict)"("Disabled"=w418) -> ()  [unwired: 2 in, 2 out]
            n476 = property on="ConnectAll" class="Bool (strict)"("Disabled"=w418) -> ()  [unwired: 2 in, 2 out]
            n477 = property on="ConnectChannel" class="Bool (strict)"("Disabled"=w418) -> ()  [unwired: 2 in, 2 out]
            n478 = property on="AddChannel" class="Bool (strict)"("Disabled"=w418) -> ()  [unwired: 2 in, 2 out]
            n479 = property on="DisconnectChannel" class="Bool (strict)"("Disabled"=w418) -> ()  [unwired: 2 in, 2 out]
            n480 = property on="ReadFromFile" class="Bool (strict)"("Disabled"=w418) -> ()  [unwired: 2 in, 2 out]
            n481 = property on="Set Output ON All" class="Bool (strict)"("Disabled"=w418) -> ()  [unwired: 2 in, 2 out]
            n482 = property on="WriteToFile" class="Bool (strict)"("Disabled"=w418) -> ()  [unwired: 2 in, 2 out]
            n483 = property on="SetOutputOnB" class="Bool (strict)"("Disabled"=w418) -> ()  [unwired: 2 in, 2 out]
            n484 = property on="CurrentModulationB" class="Bool (strict)"("Disabled"=w418) -> ()  [unwired: 2 in, 2 out]
            n485 = property on="SetCurrentB" class="Bool (strict)"("Disabled"=w418) -> ()  [unwired: 2 in, 2 out]
            n486 = property on="SetVoltageB" class="Bool (strict)"("Disabled"=w418) -> ()  [unwired: 2 in, 2 out]
            n487 = property on="SetVoltageAll" class="Bool (strict)"("Disabled"=w418) -> ()  [unwired: 2 in, 2 out]
            n488 = property on="DisconnectAll" class="Bool (strict)"("Disabled"=w418) -> ()  [unwired: 2 in, 2 out]
            n489 = property on="DeleteChannel" class="Bool (strict)"("Disabled"=w418) -> ()  [unwired: 2 in, 2 out]
            n490 = property on="SetOutputOffB" class="Bool (strict)"("Disabled"=w418) -> ()  [unwired: 2 in, 2 out]
            n491 = property on="SetCurrentAll" class="Bool (strict)"("Disabled"=w418) -> ()  [unwired: 2 in, 2 out]
          }
        }
        n492 = Merge Errors(w405) -> (w404:errorcluster)
      }
      event "SetVoltageB": Value Change {
        n493 = event-data() -> ()  [unwired: 7 out]
        n494 = local write "SetVoltageB"(FALSE ("ConnectChannel")) -> ()
        n495 = flat-sequence {
          tunnel: [w426] -> w422
          tunnel: [w435] -> w421
          tunnel: w422 -> [w435]
          frame #0 {
            w424 = u8 2 ("Disabled")
            n496 = property on="Quit" class="Bool (strict)"("Disabled"=w424) -> ()  [unwired: 2 in, 2 out]
            n497 = property on="AddChannel" class="Bool (strict)"("Disabled"=w424) -> ()  [unwired: 2 in, 2 out]
            n498 = property on="Set Output ON All" class="Bool (strict)"("Disabled"=w424) -> ()  [unwired: 2 in, 2 out]
            n499 = property on="CurrentModulationB" class="Bool (strict)"("Disabled"=w424) -> ()  [unwired: 2 in, 2 out]
            n500 = property on="ConnectAll" class="Bool (strict)"("Disabled"=w424) -> ()  [unwired: 2 in, 2 out]
            n501 = property on="DisconnectChannel" class="Bool (strict)"("Disabled"=w424) -> ()  [unwired: 2 in, 2 out]
            n502 = property on="ReadFromFile" class="Bool (strict)"("Disabled"=w424) -> ()  [unwired: 2 in, 2 out]
            n503 = property on="ConnectChannel" class="Bool (strict)"("Disabled"=w424) -> ()  [unwired: 2 in, 2 out]
            n504 = property on="DeleteChannel" class="Bool (strict)"("Disabled"=w424) -> ()  [unwired: 2 in, 2 out]
            n505 = property on="WriteToFile" class="Bool (strict)"("Disabled"=w424) -> ()  [unwired: 2 in, 2 out]
            n506 = property on="SetCurrentB" class="Bool (strict)"("Disabled"=w424) -> ()  [unwired: 2 in, 2 out]
            n507 = property on="SetOutputOnB" class="Bool (strict)"("Disabled"=w424) -> ()  [unwired: 2 in, 2 out]
            n508 = property on="SetVoltageB" class="Bool (strict)"("Disabled"=w424) -> ()  [unwired: 2 in, 2 out]
            n509 = property on="SetOutputOffB" class="Bool (strict)"("Disabled"=w424) -> ()  [unwired: 2 in, 2 out]
            n510 = property on="SetVoltageAll" class="Bool (strict)"("Disabled"=w424) -> ()  [unwired: 2 in, 2 out]
            n511 = property on="SetCurrentAll" class="Bool (strict)"("Disabled"=w424) -> ()  [unwired: 2 in, 2 out]
            n512 = property on="DisconnectAll" class="Bool (strict)"("Disabled"=w424) -> ()  [unwired: 2 in, 2 out]
          }
          frame #1 {
            n513 = property on="List of channels" class="MCListbox (strict)"() -> ("Value"=w425:i32)  [unwired: 2 in, 2 out]
            n514 = local read "VIRef"() -> (w433:refnum<vi>[])
            n515 = local read "SetVoltage"() -> (w431:dbl)
            n516 = Index Array(array=w433, index=w425) -> (element=w432:refnum<vi>)
            n517 = invoke class="VI" method="Ctrl Val.Set"(reference=w432, "Control Name"="SetVoltage", "Value"=w431) -> (reference out=w428:refnum<vi>, error out=w427:errorcluster)  [unwired: 2 in, 3 out]
            n518 = invoke class="VI" method="Ctrl Val.Set"(reference=w428, error in=w427, "Control Name"="NeedToSetVoltage", "Value"=TRUE ("ConnectChannel")) -> (error out=w426:errorcluster)  [unwired: 1 in, 4 out]
          }
          frame #2 {
            w436 = u8 0 ("Disabled")
            n519 = property on="Quit" class="Bool (strict)"("Disabled"=w436) -> ()  [unwired: 2 in, 2 out]
            n520 = property on="ConnectAll" class="Bool (strict)"("Disabled"=w436) -> ()  [unwired: 2 in, 2 out]
            n521 = property on="Set Output ON All" class="Bool (strict)"("Disabled"=w436) -> ()  [unwired: 2 in, 2 out]
            n522 = property on="AddChannel" class="Bool (strict)"("Disabled"=w436) -> ()  [unwired: 2 in, 2 out]
            n523 = property on="CurrentModulationB" class="Bool (strict)"("Disabled"=w436) -> ()  [unwired: 2 in, 2 out]
            n524 = property on="DisconnectChannel" class="Bool (strict)"("Disabled"=w436) -> ()  [unwired: 2 in, 2 out]
            n525 = property on="ReadFromFile" class="Bool (strict)"("Disabled"=w436) -> ()  [unwired: 2 in, 2 out]
            n526 = property on="ConnectChannel" class="Bool (strict)"("Disabled"=w436) -> ()  [unwired: 2 in, 2 out]
            n527 = property on="DeleteChannel" class="Bool (strict)"("Disabled"=w436) -> ()  [unwired: 2 in, 2 out]
            n528 = property on="SetVoltageAll" class="Bool (strict)"("Disabled"=w436) -> ()  [unwired: 2 in, 2 out]
            n529 = property on="SetCurrentAll" class="Bool (strict)"("Disabled"=w436) -> ()  [unwired: 2 in, 2 out]
            n530 = property on="DisconnectAll" class="Bool (strict)"("Disabled"=w436) -> ()  [unwired: 2 in, 2 out]
            n531 = property on="WriteToFile" class="Bool (strict)"("Disabled"=w436) -> ()  [unwired: 2 in, 2 out]
            n532 = property on="SetCurrentB" class="Bool (strict)"("Disabled"=w436) -> ()  [unwired: 2 in, 2 out]
            n533 = property on="SetOutputOnB" class="Bool (strict)"("Disabled"=w436) -> ()  [unwired: 2 in, 2 out]
            n534 = property on="SetVoltageB" class="Bool (strict)"("Disabled"=w436) -> ()  [unwired: 2 in, 2 out]
            n535 = property on="SetOutputOffB" class="Bool (strict)"("Disabled"=w436) -> ()  [unwired: 2 in, 2 out]
          }
        }
        n536 = Merge Errors(w421) -> (w420:errorcluster)
      }
      event "SetOutputOnB": Value Change {
        n537 = event-data() -> ()  [unwired: 2 out]
        n538 = property on="List of channels" class="MCListbox (strict)"() -> ("Value"=w440:i32)  [unwired: 2 in, 2 out]
        n539 = flat-sequence {
          tunnel: w440 -> [w442]
          tunnel: [w442] -> w439
          tunnel: w439 -> [w449]
          tunnel: [w444] -> w438
          tunnel: [w454] -> w437
          tunnel: w438 -> [w454]
          frame #0 {
            w441 = u8 2 ("Disabled")
            n540 = property on="ConnectAll" class="Bool (strict)"("Disabled"=w441) -> ()  [unwired: 2 in, 2 out]
            n541 = property on="Set Output ON All" class="Bool (strict)"("Disabled"=w441) -> ()  [unwired: 2 in, 2 out]
            n542 = property on="AddChannel" class="Bool (strict)"("Disabled"=w441) -> ()  [unwired: 2 in, 2 out]
            n543 = property on="CurrentModulationB" class="Bool (strict)"("Disabled"=w441) -> ()  [unwired: 2 in, 2 out]
            n544 = property on="DisconnectChannel" class="Bool (strict)"("Disabled"=w441) -> ()  [unwired: 2 in, 2 out]
            n545 = property on="ReadFromFile" class="Bool (strict)"("Disabled"=w441) -> ()  [unwired: 2 in, 2 out]
            n546 = property on="Quit" class="Bool (strict)"("Disabled"=w441) -> ()  [unwired: 2 in, 2 out]
            n547 = property on="ConnectChannel" class="Bool (strict)"("Disabled"=w441) -> ()  [unwired: 2 in, 2 out]
            n548 = property on="DeleteChannel" class="Bool (strict)"("Disabled"=w441) -> ()  [unwired: 2 in, 2 out]
            n549 = property on="WriteToFile" class="Bool (strict)"("Disabled"=w441) -> ()  [unwired: 2 in, 2 out]
            n550 = property on="SetCurrentB" class="Bool (strict)"("Disabled"=w441) -> ()  [unwired: 2 in, 2 out]
            n551 = property on="SetOutputOnB" class="Bool (strict)"("Disabled"=w441) -> ()  [unwired: 2 in, 2 out]
            n552 = property on="SetVoltageB" class="Bool (strict)"("Disabled"=w441) -> ()  [unwired: 2 in, 2 out]
            n553 = property on="SetOutputOffB" class="Bool (strict)"("Disabled"=w441) -> ()  [unwired: 2 in, 2 out]
            n554 = property on="SetVoltageAll" class="Bool (strict)"("Disabled"=w441) -> ()  [unwired: 2 in, 2 out]
            n555 = property on="SetCurrentAll" class="Bool (strict)"("Disabled"=w441) -> ()  [unwired: 2 in, 2 out]
            n556 = property on="DisconnectAll" class="Bool (strict)"("Disabled"=w441) -> ()  [unwired: 2 in, 2 out]
          }
          frame #1 {
            n557 = local read "VIRef"() -> (w452:refnum<vi>[])
            n558 = local write "SetOutputOnB"(FALSE ("ConnectChannel")) -> ()
            n559 = Index Array(array=w452, index=w449) -> (element=w451:refnum<vi>)
            n560 = invoke class="VI" method="Ctrl Val.Set"(reference=w451, "Control Name"="SetOutput", "Value"=TRUE ("ConnectChannel")) -> (reference out=w446:refnum<vi>, error out=w445:errorcluster)  [unwired: 2 in, 3 out]
            n561 = invoke class="VI" method="Ctrl Val.Set"(reference=w446, error in=w445, "Control Name"="NeedToSetOutput", "Value"=TRUE ("ConnectChannel")) -> (error out=w444:errorcluster)  [unwired: 1 in, 4 out]
          }
          frame #2 {
            w455 = u8 0 ("Disabled")
            n562 = property on="ConnectAll" class="Bool (strict)"("Disabled"=w455) -> ()  [unwired: 2 in, 2 out]
            n563 = property on="Set Output ON All" class="Bool (strict)"("Disabled"=w455) -> ()  [unwired: 2 in, 2 out]
            n564 = property on="AddChannel" class="Bool (strict)"("Disabled"=w455) -> ()  [unwired: 2 in, 2 out]
            n565 = property on="DisconnectChannel" class="Bool (strict)"("Disabled"=w455) -> ()  [unwired: 2 in, 2 out]
            n566 = property on="ReadFromFile" class="Bool (strict)"("Disabled"=w455) -> ()  [unwired: 2 in, 2 out]
            n567 = property on="ConnectChannel" class="Bool (strict)"("Disabled"=w455) -> ()  [unwired: 2 in, 2 out]
            n568 = property on="Quit" class="Bool (strict)"("Disabled"=w455) -> ()  [unwired: 2 in, 2 out]
            n569 = property on="DeleteChannel" class="Bool (strict)"("Disabled"=w455) -> ()  [unwired: 2 in, 2 out]
            n570 = property on="SetOutputOffB" class="Bool (strict)"("Disabled"=w455) -> ()  [unwired: 2 in, 2 out]
            n571 = property on="CurrentModulationB" class="Bool (strict)"("Disabled"=w455) -> ()  [unwired: 2 in, 2 out]
            n572 = property on="SetVoltageAll" class="Bool (strict)"("Disabled"=w455) -> ()  [unwired: 2 in, 2 out]
            n573 = property on="SetCurrentAll" class="Bool (strict)"("Disabled"=w455) -> ()  [unwired: 2 in, 2 out]
            n574 = property on="DisconnectAll" class="Bool (strict)"("Disabled"=w455) -> ()  [unwired: 2 in, 2 out]
            n575 = property on="WriteToFile" class="Bool (strict)"("Disabled"=w455) -> ()  [unwired: 2 in, 2 out]
            n576 = property on="SetCurrentB" class="Bool (strict)"("Disabled"=w455) -> ()  [unwired: 2 in, 2 out]
            n577 = property on="SetOutputOnB" class="Bool (strict)"("Disabled"=w455) -> ()  [unwired: 2 in, 2 out]
            n578 = property on="SetVoltageB" class="Bool (strict)"("Disabled"=w455) -> ()  [unwired: 2 in, 2 out]
          }
        }
      }
      event "Set Output ON All": Value Change {
        n579 = event-data() -> ("NewVal"=w456:bool)  [unwired: 1 out]
        n580 = flat-sequence {
          tunnel: [w461] -> w457
          tunnel: w456 -> [w461]
          tunnel: [w466] -> w459
          tunnel: w457 -> [w463]
          tunnel: [w477] -> w460
          tunnel: w459 -> [w477]
          frame #0 {
            w462 = u8 2 ("Disabled")
            n581 = property on="Quit" class="Bool (strict)"("Disabled"=w462) -> ()  [unwired: 2 in, 2 out]
            n582 = property on="AddChannel" class="Bool (strict)"("Disabled"=w462) -> ()  [unwired: 2 in, 2 out]
            n583 = property on="CurrentModulationB" class="Bool (strict)"("Disabled"=w462) -> ()  [unwired: 2 in, 2 out]
            n584 = property on="DisconnectChannel" class="Bool (strict)"("Disabled"=w462) -> ()  [unwired: 2 in, 2 out]
            n585 = property on="ConnectAll" class="Bool (strict)"("Disabled"=w462) -> ()  [unwired: 2 in, 2 out]
            n586 = property on="ReadFromFile" class="Bool (strict)"("Disabled"=w462) -> ()  [unwired: 2 in, 2 out]
            n587 = property on="ConnectChannel" class="Bool (strict)"("Disabled"=w462) -> ()  [unwired: 2 in, 2 out]
            n588 = property on="DeleteChannel" class="Bool (strict)"("Disabled"=w462) -> ()  [unwired: 2 in, 2 out]
            n589 = property on="WriteToFile" class="Bool (strict)"("Disabled"=w462) -> ()  [unwired: 2 in, 2 out]
            n590 = property on="SetCurrentB" class="Bool (strict)"("Disabled"=w462) -> ()  [unwired: 2 in, 2 out]
            n591 = property on="SetOutputOnB" class="Bool (strict)"("Disabled"=w462) -> ()  [unwired: 2 in, 2 out]
            n592 = property on="SetVoltageB" class="Bool (strict)"("Disabled"=w462) -> ()  [unwired: 2 in, 2 out]
            n593 = property on="SetOutputOffB" class="Bool (strict)"("Disabled"=w462) -> ()  [unwired: 2 in, 2 out]
            n594 = property on="SetVoltageAll" class="Bool (strict)"("Disabled"=w462) -> ()  [unwired: 2 in, 2 out]
            n595 = property on="SetCurrentAll" class="Bool (strict)"("Disabled"=w462) -> ()  [unwired: 2 in, 2 out]
            n596 = property on="DisconnectAll" class="Bool (strict)"("Disabled"=w462) -> ()  [unwired: 2 in, 2 out]
          }
          frame #1 {
            n597 = local read "VIRef"() -> (w465:refnum<vi>[])
            n598 = Array Size(array=w465) -> (size(s)=w464:i32)
            n599 = for {
              N: w464 -> [_]
              tunnel: [w468] -> w466 mode=indexing
              tunnel: w463 -> [w467]
              i -> [w470]
              n600 = local read "VIRef"() -> (w475:refnum<vi>[])
              n601 = Index Array(array=w475, index=w470) -> (element=w474:refnum<vi>)
              n602 = invoke class="VI" method="Ctrl Val.Set"(reference=w474, "Control Name"="SetOutput", "Value"=w467) -> (reference out=w471:refnum<vi>, error out=w469:errorcluster)  [unwired: 2 in, 3 out]
              n603 = invoke class="VI" method="Ctrl Val.Set"(reference=w471, error in=w469, "Control Name"="NeedToSetOutput", "Value"=TRUE ("ConnectChannel")) -> (error out=w468:errorcluster)  [unwired: 1 in, 4 out]
            }
          }
          frame #2 {
            w478 = u8 0 ("Disabled")
            n604 = disable-structure shown="Disabled" {
              frame Disabled {
                n605 = local write "Set Output ON All"(FALSE ("ConnectChannel")) -> ()
              }
              frame Enabled {
              }
            }
            n606 = property on="Quit" class="Bool (strict)"("Disabled"=w478) -> ()  [unwired: 2 in, 2 out]
            n607 = property on="ConnectAll" class="Bool (strict)"("Disabled"=w478) -> ()  [unwired: 2 in, 2 out]
            n608 = property on="Set Output ON All" class="Bool (strict)"("Disabled"=w478) -> ()  [unwired: 2 in, 2 out]
            n609 = property on="AddChannel" class="Bool (strict)"("Disabled"=w478) -> ()  [unwired: 2 in, 2 out]
            n610 = property on="DisconnectChannel" class="Bool (strict)"("Disabled"=w478) -> ()  [unwired: 2 in, 2 out]
            n611 = property on="ReadFromFile" class="Bool (strict)"("Disabled"=w478) -> ()  [unwired: 2 in, 2 out]
            n612 = property on="ConnectChannel" class="Bool (strict)"("Disabled"=w478) -> ()  [unwired: 2 in, 2 out]
            n613 = property on="DeleteChannel" class="Bool (strict)"("Disabled"=w478) -> ()  [unwired: 2 in, 2 out]
            n614 = property on="SetVoltageB" class="Bool (strict)"("Disabled"=w478) -> ()  [unwired: 2 in, 2 out]
            n615 = property on="CurrentModulationB" class="Bool (strict)"("Disabled"=w478) -> ()  [unwired: 2 in, 2 out]
            n616 = property on="SetOutputOffB" class="Bool (strict)"("Disabled"=w478) -> ()  [unwired: 2 in, 2 out]
            n617 = property on="SetVoltageAll" class="Bool (strict)"("Disabled"=w478) -> ()  [unwired: 2 in, 2 out]
            n618 = property on="SetCurrentAll" class="Bool (strict)"("Disabled"=w478) -> ()  [unwired: 2 in, 2 out]
            n619 = property on="DisconnectAll" class="Bool (strict)"("Disabled"=w478) -> ()  [unwired: 2 in, 2 out]
            n620 = property on="WriteToFile" class="Bool (strict)"("Disabled"=w478) -> ()  [unwired: 2 in, 2 out]
            n621 = property on="SetCurrentB" class="Bool (strict)"("Disabled"=w478) -> ()  [unwired: 2 in, 2 out]
            n622 = property on="SetOutputOnB" class="Bool (strict)"("Disabled"=w478) -> ()  [unwired: 2 in, 2 out]
          }
        }
        n623 = Merge Errors(w460) -> (w458:errorcluster)
      }
      event "SetOutputOffB": Value Change {
        n624 = event-data() -> ()  [unwired: 7 out]
        n625 = local write "SetOutputOffB"(FALSE ("ConnectChannel")) -> ()
        n626 = property on="List of channels" class="MCListbox (strict)"() -> ("Value"=w484:i32)  [unwired: 2 in, 2 out]
        n627 = flat-sequence {
          tunnel: w484 -> [w486]
          tunnel: [w486] -> w483
          tunnel: w483 -> [w493]
          tunnel: [w487] -> w480
          tunnel: [w497] -> w481
          tunnel: w480 -> [w497]
          frame #0 {
            w485 = u8 2 ("Disabled")
            n628 = property on="ConnectAll" class="Bool (strict)"("Disabled"=w485) -> ()  [unwired: 2 in, 2 out]
            n629 = property on="Set Output ON All" class="Bool (strict)"("Disabled"=w485) -> ()  [unwired: 2 in, 2 out]
            n630 = property on="AddChannel" class="Bool (strict)"("Disabled"=w485) -> ()  [unwired: 2 in, 2 out]
            n631 = property on="CurrentModulationB" class="Bool (strict)"("Disabled"=w485) -> ()  [unwired: 2 in, 2 out]
            n632 = property on="DisconnectChannel" class="Bool (strict)"("Disabled"=w485) -> ()  [unwired: 2 in, 2 out]
            n633 = property on="ReadFromFile" class="Bool (strict)"("Disabled"=w485) -> ()  [unwired: 2 in, 2 out]
            n634 = property on="Quit" class="Bool (strict)"("Disabled"=w485) -> ()  [unwired: 2 in, 2 out]
            n635 = property on="ConnectChannel" class="Bool (strict)"("Disabled"=w485) -> ()  [unwired: 2 in, 2 out]
            n636 = property on="DeleteChannel" class="Bool (strict)"("Disabled"=w485) -> ()  [unwired: 2 in, 2 out]
            n637 = property on="WriteToFile" class="Bool (strict)"("Disabled"=w485) -> ()  [unwired: 2 in, 2 out]
            n638 = property on="SetCurrentB" class="Bool (strict)"("Disabled"=w485) -> ()  [unwired: 2 in, 2 out]
            n639 = property on="SetOutputOnB" class="Bool (strict)"("Disabled"=w485) -> ()  [unwired: 2 in, 2 out]
            n640 = property on="SetVoltageB" class="Bool (strict)"("Disabled"=w485) -> ()  [unwired: 2 in, 2 out]
            n641 = property on="SetOutputOffB" class="Bool (strict)"("Disabled"=w485) -> ()  [unwired: 2 in, 2 out]
            n642 = property on="SetVoltageAll" class="Bool (strict)"("Disabled"=w485) -> ()  [unwired: 2 in, 2 out]
            n643 = property on="SetCurrentAll" class="Bool (strict)"("Disabled"=w485) -> ()  [unwired: 2 in, 2 out]
            n644 = property on="DisconnectAll" class="Bool (strict)"("Disabled"=w485) -> ()  [unwired: 2 in, 2 out]
          }
          frame #1 {
            n645 = local read "VIRef"() -> (w495:refnum<vi>[])
            n646 = Index Array(array=w495, index=w493) -> (element=w494:refnum<vi>)
            n647 = invoke class="VI" method="Ctrl Val.Set"(reference=w494, "Control Name"="SetOutput", "Value"=FALSE ("ConnectChannel")) -> (reference out=w490:refnum<vi>, error out=w488:errorcluster)  [unwired: 2 in, 3 out]
            n648 = invoke class="VI" method="Ctrl Val.Set"(reference=w490, error in=w488, "Control Name"="NeedToSetOutput", "Value"=TRUE ("ConnectChannel")) -> (error out=w487:errorcluster)  [unwired: 1 in, 4 out]
          }
          frame #2 {
            w498 = u8 0 ("Disabled")
            n649 = property on="ConnectAll" class="Bool (strict)"("Disabled"=w498) -> ()  [unwired: 2 in, 2 out]
            n650 = property on="Set Output ON All" class="Bool (strict)"("Disabled"=w498) -> ()  [unwired: 2 in, 2 out]
            n651 = property on="AddChannel" class="Bool (strict)"("Disabled"=w498) -> ()  [unwired: 2 in, 2 out]
            n652 = property on="CurrentModulationB" class="Bool (strict)"("Disabled"=w498) -> ()  [unwired: 2 in, 2 out]
            n653 = property on="DisconnectChannel" class="Bool (strict)"("Disabled"=w498) -> ()  [unwired: 2 in, 2 out]
            n654 = property on="ReadFromFile" class="Bool (strict)"("Disabled"=w498) -> ()  [unwired: 2 in, 2 out]
            n655 = property on="ConnectChannel" class="Bool (strict)"("Disabled"=w498) -> ()  [unwired: 2 in, 2 out]
            n656 = property on="Quit" class="Bool (strict)"("Disabled"=w498) -> ()  [unwired: 2 in, 2 out]
            n657 = property on="DeleteChannel" class="Bool (strict)"("Disabled"=w498) -> ()  [unwired: 2 in, 2 out]
            n658 = property on="SetOutputOffB" class="Bool (strict)"("Disabled"=w498) -> ()  [unwired: 2 in, 2 out]
            n659 = property on="SetVoltageAll" class="Bool (strict)"("Disabled"=w498) -> ()  [unwired: 2 in, 2 out]
            n660 = property on="SetCurrentAll" class="Bool (strict)"("Disabled"=w498) -> ()  [unwired: 2 in, 2 out]
            n661 = property on="DisconnectAll" class="Bool (strict)"("Disabled"=w498) -> ()  [unwired: 2 in, 2 out]
            n662 = property on="WriteToFile" class="Bool (strict)"("Disabled"=w498) -> ()  [unwired: 2 in, 2 out]
            n663 = property on="SetCurrentB" class="Bool (strict)"("Disabled"=w498) -> ()  [unwired: 2 in, 2 out]
            n664 = property on="SetOutputOnB" class="Bool (strict)"("Disabled"=w498) -> ()  [unwired: 2 in, 2 out]
            n665 = property on="SetVoltageB" class="Bool (strict)"("Disabled"=w498) -> ()  [unwired: 2 in, 2 out]
          }
        }
      }
      event "WriteToFile": Value Change {
        n666 = event-data() -> ()  [unwired: 7 out]
        n667 = local read "ADRESS"() -> (w503:string[])
        n668 = Array Size(array=w503) -> (size(s)=w502:i32)
        n669 = flat-sequence {
          tunnel: w502 -> [w512]
          tunnel: [w504] -> w500
          tunnel: [w545] -> w501
          tunnel: w500 -> [w545]
          frame #0 {
            n670 = Number To Decimal String(number=w512) -> (decimal integer string=w507:string)  [unwired: 1 out]
            n671 = Write to Text File(text=w507) -> (refnum out=w506:refnum<file>, cancelled=w505:bool, error out=w508:errorcluster)  [unwired: 1 in, 2 out]
            n672 = Write to Text File(file (use dialog)=w506, text="\nИМЯ  АДРЕС  ТОК  НАПРЯЖЕНИЕ", error in=w508) -> (refnum out=w509:refnum<file>, error out=w510:errorcluster)  [unwired: 2 out]
            n673 = for {
              N: w512 -> [_]
              tunnel: w505 -> [w522]
              tunnel: w510 -> [w517]
              tunnel: w509 -> [w524]
              tunnel: [w515] -> w504 mode=indexing
              i -> [w523]
              w528 = "" ("Control Name")
              w534 = "\t"
              n674 = local read "VIRef"() -> (w532:refnum<vi>[])
              n675 = Index Array(array=w532, index=w523) -> (element=w531:refnum<vi>)
              n676 = invoke class="VI" method="Ctrl Val.Get"(reference=w531, "Control Name"="SetVoltageStr") -> (reference out=w526:refnum<vi>, error out=w519:errorcluster, "Get Control Value Variant"=w533:variant)  [unwired: 2 in, 1 out]
              n677 = invoke class="VI" method="Ctrl Val.Get"(reference=w526, error in=w519, "Control Name"="SetCurrentStr") -> (error out=w518:errorcluster, "Get Control Value Variant"=w529:variant)  [unwired: 1 in, 2 out]
              n678 = local read "ADRESS"() -> (w539:string[])
              n679 = local read "NAME"() -> (w537:string[])
              n680 = Index Array(array=w537, index=w523) -> (element=w535:string)
              n681 = Index Array(array=w539, index=w523) -> (element=w538:string)
              n682 = Variant To Data(type=w528, Variant=w529) -> (data=w514:string, error out=w521:errorcluster)  [unwired: 1 in]
              n683 = Variant To Data(type=w528, Variant=w533) -> (data=w513:string, error out=w520:errorcluster)  [unwired: 1 in]
              n684 = Merge Errors(w518, w521, w520, w517) -> (w516:errorcluster)
              n685 = Concatenate Strings("\r\n", w535, w534, w538, w534, w514, w534, w513) -> (w525:string)
              n686 = case shown="True" w522 {
                tunnel: w524 -> [w542 _]
                tunnel: w525 -> [w543 _]
                tunnel: w516 -> [w541 w544]
                tunnel: [w540 w544] -> w515
                frame False {
                  n687 = Write to Text File(file (use dialog)=w542, text=w543, error in=w541) -> (error out=w540:errorcluster)  [unwired: 3 out]
                }
                frame True {
                }
              }
            }
          }
          frame #1 {
            n688 = local write "WriteToFile"(FALSE ("ConnectChannel")) -> ()
          }
        }
        n689 = Merge Errors(w501) -> (w499:errorcluster)
      }
      event "ReadFromFile": Value Change {
        n690 = event-data() -> ()  [unwired: 2 out]
        n691 = local read "ReadFromFile"() -> (w549:bool)
        n692 = Read from Text File(count=100) -> (text=w553:string[], cancelled=w552:bool, error out=w551:errorcluster)  [unwired: 1 in, 3 out]
        n693 = Not(x=w552) -> (.not. x?=w548:bool)
        n694 = And(x=w549, y=w548) -> (x .and. y?=w547:bool)
        n695 = case shown="True" w547 {
          tunnel: w553 -> [_ w557]
          tunnel: w551 -> [w555 w559]
          tunnel: [w555 w558] -> w550
          frame False {
            n696 = local write "ReadFromFile"(FALSE ("ConnectChannel")) -> ()
          }
          frame True {
            n697 = flat-sequence {
              tunnel: w559 -> [w567]
              tunnel: [w566] -> w561
              tunnel: w561 -> [w576]
              tunnel: [w576] -> w560
              tunnel: w560 -> [_]
              tunnel: [w587] -> w563
              tunnel: w557 -> [w586]
              tunnel: w563 -> [w621]
              tunnel: [w621] -> w562
              frame #0 {
                w565 = u8 2 ("Disabled")
                n698 = local read "VIRef"() -> (w568:refnum<vi>[])
                n699 = property on="Set Output ON All" class="Bool (strict)"("Disabled"=w565) -> ()  [unwired: 2 in, 2 out]
                n700 = property on="CurrentModulationB" class="Bool (strict)"("Disabled"=w565) -> ()  [unwired: 2 in, 2 out]
                n701 = property on="ConnectAll" class="Bool (strict)"("Disabled"=w565) -> ()  [unwired: 2 in, 2 out]
                n702 = property on="ReadFromFile" class="Bool (strict)"("Disabled"=w565) -> ()  [unwired: 2 in, 2 out]
                n703 = property on="ConnectChannel" class="Bool (strict)"("Disabled"=w565) -> ()  [unwired: 2 in, 2 out]
                n704 = property on="DisconnectChannel" class="Bool (strict)"("Disabled"=w565) -> ()  [unwired: 2 in, 2 out]
                n705 = property on="WriteToFile" class="Bool (strict)"("Disabled"=w565) -> ()  [unwired: 2 in, 2 out]
                n706 = property on="AddChannel" class="Bool (strict)"("Disabled"=w565) -> ()  [unwired: 2 in, 2 out]
                n707 = property on="SetOutputOnB" class="Bool (strict)"("Disabled"=w565) -> ()  [unwired: 2 in, 2 out]
                n708 = property on="Quit" class="Bool (strict)"("Disabled"=w565) -> ()  [unwired: 2 in, 2 out]
                n709 = property on="DeleteChannel" class="Bool (strict)"("Disabled"=w565) -> ()  [unwired: 2 in, 2 out]
                n710 = property on="SetCurrentB" class="Bool (strict)"("Disabled"=w565) -> ()  [unwired: 2 in, 2 out]
                n711 = property on="SetOutputOffB" class="Bool (strict)"("Disabled"=w565) -> ()  [unwired: 2 in, 2 out]
                n712 = property on="SetCurrentAll" class="Bool (strict)"("Disabled"=w565) -> ()  [unwired: 2 in, 2 out]
                n713 = property on="SetVoltageB" class="Bool (strict)"("Disabled"=w565) -> ()  [unwired: 2 in, 2 out]
                n714 = property on="SetVoltageAll" class="Bool (strict)"("Disabled"=w565) -> ()  [unwired: 2 in, 2 out]
                n715 = property on="DisconnectAll" class="Bool (strict)"("Disabled"=w565) -> ()  [unwired: 2 in, 2 out]
                n716 = Array Size(array=w568) -> (size(s)=w564:i32)
                n717 = for {
                  N: w564 -> [_]
                  tunnel: w568 -> [w572]
                  tunnel: w567 -> [w570]
                  tunnel: [w569] -> w566 mode=indexing
                  i -> [w573]
                  n718 = Index Array(array=w572, index=w573) -> (element=w571:refnum<vi>)
                  n719 = invoke class="VI" method="Ctrl Val.Set"(reference=w571, error in=w570, "Control Name"="Connect", "Value"=FALSE) -> (error out=w569:errorcluster)  [unwired: 1 in, 4 out]
                }
              }
              frame #1 {
                n720 = Wait (ms)(milliseconds to wait=u32 1000) -> ()  [unwired: 1 out]
              }
              frame #2 {
                n721 = local read "VIRef"() -> (w579:refnum<vi>[])
                n722 = Array Size(array=w579) -> (size(s)=w578:i32)
                n723 = for {
                  N: w578 -> [_]
                  tunnel: w579 -> [w581]
                  i -> [w582]
                  n724 = Index Array(array=w581, index=w582) -> (element=w580:refnum<vi>)
                  n725 = invoke class="VI" method="Abort VI"(reference=w580) -> ()  [unwired: 2 in, 3 out]
                }
              }
              frame #3 {
                w584 = string[] [] ("GlobalInAdress")
                n726 = Wait (ms)(milliseconds to wait=u32 250) -> ()  [unwired: 1 out]
                n727 = local write "NAME"(w584) -> ()
                n728 = local write "ADRESS"(w584) -> ()
                n729 = local write "VIRef"(refnum<vi>[] []) -> ()
              }
              frame #4 {
                n730 = Index Array(array=w586, index=0) -> (element=w590:string)
                n731 = Decimal String To Number(string=w590) -> (number=w588:i32)  [unwired: 3 out]
                n732 = for {
                  N: w588 -> [_]
                  tunnel: w586 -> [w615]
                  tunnel: [w591] -> w587 mode=indexing
                  i -> [w618]
                  n733 = Add(x=2, y=w618) -> (x+y=w617:i32)
                  n734 = Index Array(array=w615, index=w617) -> (element=w614:string)
                  n735 = Spreadsheet String To Array(format string="%s", spreadsheet string=w614, array type (2D Dbl)=string[] [] ("GlobalInAdress")) -> (array=w605:string[])  [unwired: 1 out]
                  n736 = Index Array(array=w605, index=3) -> (element=w603:string)
                  n737 = Index Array(array=w605, index=0) -> (element=w609:string)
                  n738 = Index Array(array=w605, index=1) -> (element=w610:string)
                  n739 = Index Array(array=w605, index=2) -> (element=w604:string)
                  n740 = local read "ADRESS"() -> (w601:string[])
                  n741 = Scan From String(input string=w603, default 1=0.0 ("default value 1")) -> (output 1=w596:dbl)  [unwired: 3 in, 3 out]
                  n742 = Scan From String(input string=w604, default 1=0.0 ("default value 1")) -> (output 1=w598:dbl)  [unwired: 3 in, 3 out]
                  n743 = local read "NAME"() -> (w602:string[])
                  n744 = local read "VIRef"() -> (w600:refnum<vi>[])
                  n745 = call "AddChannel.vi"("VIRef"=w600, "Name"=w609, "SetCurrent"=w596, "ADRESS"=w601, "NAME"=w602, "Address"=w610, "SetVoltage"=w598) -> ("NAMEOut"=w595:string[], "error out"=w592:errorcluster, "ADRESSOut"=w593:string[], "VIRefOut"=w594:refnum<vi>[])  [unwired: 1 in, 4 out]
                  n746 = local write "NAME"(w595) -> ()
                  n747 = local write "VIRef"(w594) -> ()
                  n748 = flat-sequence {
                    tunnel: w592 -> [w620]
                    tunnel: [w620] -> w591
                    frame #0 {
                      n749 = Wait (ms)(milliseconds to wait=u32 50) -> ()  [unwired: 1 out]
                    }
                  }
                  n750 = local write "ADRESS"(w593) -> ()
                }
              }
              frame #5 {
                w622 = u8 0 ("Disabled")
                n751 = local write "ReadFromFile"(FALSE ("ConnectChannel")) -> ()
                n752 = property on="ConnectAll" class="Bool (strict)"("Disabled"=w622) -> ()  [unwired: 2 in, 2 out]
                n753 = property on="Set Output ON All" class="Bool (strict)"("Disabled"=w622) -> ()  [unwired: 2 in, 2 out]
                n754 = property on="AddChannel" class="Bool (strict)"("Disabled"=w622) -> ()  [unwired: 2 in, 2 out]
                n755 = property on="CurrentModulationB" class="Bool (strict)"("Disabled"=w622) -> ()  [unwired: 2 in, 2 out]
                n756 = property on="DisconnectChannel" class="Bool (strict)"("Disabled"=w622) -> ()  [unwired: 2 in, 2 out]
                n757 = property on="ReadFromFile" class="Bool (strict)"("Disabled"=w622) -> ()  [unwired: 2 in, 2 out]
                n758 = property on="ConnectChannel" class="Bool (strict)"("Disabled"=w622) -> ()  [unwired: 2 in, 2 out]
                n759 = property on="DeleteChannel" class="Bool (strict)"("Disabled"=w622) -> ()  [unwired: 2 in, 2 out]
                n760 = property on="WriteToFile" class="Bool (strict)"("Disabled"=w622) -> ()  [unwired: 2 in, 2 out]
                n761 = property on="SetCurrentB" class="Bool (strict)"("Disabled"=w622) -> ()  [unwired: 2 in, 2 out]
                n762 = property on="Quit" class="Bool (strict)"("Disabled"=w622) -> ()  [unwired: 2 in, 2 out]
                n763 = property on="SetOutputOnB" class="Bool (strict)"("Disabled"=w622) -> ()  [unwired: 2 in, 2 out]
                n764 = property on="SetVoltageB" class="Bool (strict)"("Disabled"=w622) -> ()  [unwired: 2 in, 2 out]
                n765 = property on="SetOutputOffB" class="Bool (strict)"("Disabled"=w622) -> ()  [unwired: 2 in, 2 out]
                n766 = property on="SetVoltageAll" class="Bool (strict)"("Disabled"=w622) -> ()  [unwired: 2 in, 2 out]
                n767 = property on="SetCurrentAll" class="Bool (strict)"("Disabled"=w622) -> ()  [unwired: 2 in, 2 out]
                n768 = property on="DisconnectAll" class="Bool (strict)"("Disabled"=w622) -> ()  [unwired: 2 in, 2 out]
              }
            }
            n769 = Merge Errors(w562) -> (w558:errorcluster)
          }
        }
      }
      event "SetCurrentB": Value Change {
        n770 = event-data() -> ()  [unwired: 7 out]
        n771 = local write "SetCurrentB"(FALSE ("ConnectChannel")) -> ()
        n772 = property on="List of channels" class="MCListbox (strict)"() -> (error out=w626:errorcluster, "Value"=w630:i32)  [unwired: 2 in, 1 out]
        n773 = flat-sequence {
          tunnel: w630 -> [w633]
          tunnel: [w633] -> w629
          tunnel: [w631] -> w627
          tunnel: w626 -> [w631]
          tunnel: w629 -> [w635]
          tunnel: w627 -> [w634]
          tunnel: [w636] -> w625
          tunnel: [w645] -> w624
          tunnel: w625 -> [w645]
          frame #0 {
            w632 = u8 2 ("Disabled")
            n774 = property on="AddChannel" class="Bool (strict)"("Disabled"=w632) -> ()  [unwired: 2 in, 2 out]
            n775 = property on="Set Output ON All" class="Bool (strict)"("Disabled"=w632) -> ()  [unwired: 2 in, 2 out]
            n776 = property on="CurrentModulationB" class="Bool (strict)"("Disabled"=w632) -> ()  [unwired: 2 in, 2 out]
            n777 = property on="ConnectAll" class="Bool (strict)"("Disabled"=w632) -> ()  [unwired: 2 in, 2 out]
            n778 = property on="DisconnectChannel" class="Bool (strict)"("Disabled"=w632) -> ()  [unwired: 2 in, 2 out]
            n779 = property on="ReadFromFile" class="Bool (strict)"("Disabled"=w632) -> ()  [unwired: 2 in, 2 out]
            n780 = property on="Quit" class="Bool (strict)"("Disabled"=w632) -> ()  [unwired: 2 in, 2 out]
            n781 = property on="ConnectChannel" class="Bool (strict)"("Disabled"=w632) -> ()  [unwired: 2 in, 2 out]
            n782 = property on="DeleteChannel" class="Bool (strict)"("Disabled"=w632) -> ()  [unwired: 2 in, 2 out]
            n783 = property on="WriteToFile" class="Bool (strict)"("Disabled"=w632) -> ()  [unwired: 2 in, 2 out]
            n784 = property on="SetCurrentB" class="Bool (strict)"("Disabled"=w632) -> ()  [unwired: 2 in, 2 out]
            n785 = property on="SetOutputOnB" class="Bool (strict)"("Disabled"=w632) -> ()  [unwired: 2 in, 2 out]
            n786 = property on="SetVoltageB" class="Bool (strict)"("Disabled"=w632) -> ()  [unwired: 2 in, 2 out]
            n787 = property on="SetOutputOffB" class="Bool (strict)"("Disabled"=w632) -> ()  [unwired: 2 in, 2 out]
            n788 = property on="SetVoltageAll" class="Bool (strict)"("Disabled"=w632) -> ()  [unwired: 2 in, 2 out]
            n789 = property on="SetCurrentAll" class="Bool (strict)"("Disabled"=w632) -> ()  [unwired: 2 in, 2 out]
            n790 = property on="DisconnectAll" class="Bool (strict)"("Disabled"=w632) -> ()  [unwired: 2 in, 2 out]
          }
          frame #1 {
            n791 = local read "VIRef"() -> (w643:refnum<vi>[])
            n792 = local read "SetCurrent"() -> (w641:dbl)
            n793 = Index Array(array=w643, index=w635) -> (element=w642:refnum<vi>)
            n794 = invoke class="VI" method="Ctrl Val.Set"(reference=w642, error in=w634, "Control Name"="SetCurrent", "Value"=w641) -> (reference out=w638:refnum<vi>, error out=w637:errorcluster)  [unwired: 1 in, 3 out]
            n795 = invoke class="VI" method="Ctrl Val.Set"(reference=w638, error in=w637, "Control Name"="NeedToSetCurrent", "Value"=TRUE ("ConnectChannel")) -> (error out=w636:errorcluster)  [unwired: 1 in, 4 out]
          }
          frame #2 {
            w646 = u8 0 ("Disabled")
            n796 = property on="AddChannel" class="Bool (strict)"("Disabled"=w646) -> ()  [unwired: 2 in, 2 out]
            n797 = property on="Set Output ON All" class="Bool (strict)"("Disabled"=w646) -> ()  [unwired: 2 in, 2 out]
            n798 = property on="DisconnectChannel" class="Bool (strict)"("Disabled"=w646) -> ()  [unwired: 2 in, 2 out]
            n799 = property on="ConnectAll" class="Bool (strict)"("Disabled"=w646) -> ()  [unwired: 2 in, 2 out]
            n800 = property on="ReadFromFile" class="Bool (strict)"("Disabled"=w646) -> ()  [unwired: 2 in, 2 out]
            n801 = property on="ConnectChannel" class="Bool (strict)"("Disabled"=w646) -> ()  [unwired: 2 in, 2 out]
            n802 = property on="DeleteChannel" class="Bool (strict)"("Disabled"=w646) -> ()  [unwired: 2 in, 2 out]
            n803 = property on="Quit" class="Bool (strict)"("Disabled"=w646) -> ()  [unwired: 2 in, 2 out]
            n804 = property on="WriteToFile" class="Bool (strict)"("Disabled"=w646) -> ()  [unwired: 2 in, 2 out]
            n805 = property on="CurrentModulationB" class="Bool (strict)"("Disabled"=w646) -> ()  [unwired: 2 in, 2 out]
            n806 = property on="SetCurrentB" class="Bool (strict)"("Disabled"=w646) -> ()  [unwired: 2 in, 2 out]
            n807 = property on="SetOutputOnB" class="Bool (strict)"("Disabled"=w646) -> ()  [unwired: 2 in, 2 out]
            n808 = property on="SetVoltageB" class="Bool (strict)"("Disabled"=w646) -> ()  [unwired: 2 in, 2 out]
            n809 = property on="SetOutputOffB" class="Bool (strict)"("Disabled"=w646) -> ()  [unwired: 2 in, 2 out]
            n810 = property on="SetVoltageAll" class="Bool (strict)"("Disabled"=w646) -> ()  [unwired: 2 in, 2 out]
            n811 = property on="SetCurrentAll" class="Bool (strict)"("Disabled"=w646) -> ()  [unwired: 2 in, 2 out]
            n812 = property on="DisconnectAll" class="Bool (strict)"("Disabled"=w646) -> ()  [unwired: 2 in, 2 out]
          }
        }
      }
      event "DeleteChannel": Value Change {
        n813 = event-data() -> ()  [unwired: 7 out]
        n814 = property on="List of channels" class="MCListbox (strict)"() -> ("Value"=w650:i32)  [unwired: 2 in, 2 out]
        n815 = flat-sequence {
          tunnel: [w659] -> w651
          tunnel: w650 -> [w659]
          tunnel: [w663] -> w658
          tunnel: [w661] -> w657
          tunnel: [w662] -> w656
          tunnel: w651 -> [w661]
          tunnel: [w669] -> w655
          tunnel: w658 -> [w669]
          tunnel: [w668] -> w654
          tunnel: w657 -> [w668]
          tunnel: w656 -> [w667]
          tunnel: [w667] -> w653
          tunnel: w655 -> [w674]
          tunnel: [w673] -> w652
          tunnel: w654 -> [w673]
          tunnel: w653 -> [w672]
          tunnel: [w671] -> w648
          tunnel: w652 -> [w676]
          tunnel: [w675] -> w649
          tunnel: w648 -> [w675]
          tunnel: w649 -> [w684]
          tunnel: [w684] -> w647
          frame #0 {
            w660 = u8 2 ("Disabled")
            n816 = property on="AddChannel" class="Bool (strict)"("Disabled"=w660) -> ()  [unwired: 2 in, 2 out]
            n817 = property on="Set Output ON All" class="Bool (strict)"("Disabled"=w660) -> ()  [unwired: 2 in, 2 out]
            n818 = property on="CurrentModulationB" class="Bool (strict)"("Disabled"=w660) -> ()  [unwired: 2 in, 2 out]
            n819 = property on="ConnectAll" class="Bool (strict)"("Disabled"=w660) -> ()  [unwired: 2 in, 2 out]
            n820 = property on="DisconnectChannel" class="Bool (strict)"("Disabled"=w660) -> ()  [unwired: 2 in, 2 out]
            n821 = property on="ReadFromFile" class="Bool (strict)"("Disabled"=w660) -> ()  [unwired: 2 in, 2 out]
            n822 = property on="Quit" class="Bool (strict)"("Disabled"=w660) -> ()  [unwired: 2 in, 2 out]
            n823 = property on="ConnectChannel" class="Bool (strict)"("Disabled"=w660) -> ()  [unwired: 2 in, 2 out]
            n824 = property on="DeleteChannel" class="Bool (strict)"("Disabled"=w660) -> ()  [unwired: 2 in, 2 out]
            n825 = property on="WriteToFile" class="Bool (strict)"("Disabled"=w660) -> ()  [unwired: 2 in, 2 out]
            n826 = property on="SetCurrentB" class="Bool (strict)"("Disabled"=w660) -> ()  [unwired: 2 in, 2 out]
            n827 = property on="SetOutputOnB" class="Bool (strict)"("Disabled"=w660) -> ()  [unwired: 2 in, 2 out]
            n828 = property on="SetVoltageB" class="Bool (strict)"("Disabled"=w660) -> ()  [unwired: 2 in, 2 out]
            n829 = property on="SetOutputOffB" class="Bool (strict)"("Disabled"=w660) -> ()  [unwired: 2 in, 2 out]
            n830 = property on="SetVoltageAll" class="Bool (strict)"("Disabled"=w660) -> ()  [unwired: 2 in, 2 out]
            n831 = property on="SetCurrentAll" class="Bool (strict)"("Disabled"=w660) -> ()  [unwired: 2 in, 2 out]
            n832 = property on="DisconnectAll" class="Bool (strict)"("Disabled"=w660) -> ()  [unwired: 2 in, 2 out]
          }
          frame #1 {
            n833 = local read "VIRef"() -> (w665:refnum<vi>[])
            n834 = Index Array(array=w665, index=w661) -> (element=w663:refnum<vi>)
            n835 = invoke class="VI" method="Ctrl Val.Set"(reference=w663, "Control Name"="Connect", "Value"=FALSE ("OK Button")) -> (error out=w662:errorcluster)  [unwired: 2 in, 4 out]
          }
          frame #2 {
            n836 = Wait (ms)(milliseconds to wait=u32 1000) -> ()  [unwired: 1 out]
          }
          frame #3 {
            n837 = invoke class="VI" method="Abort VI"(reference=w674, error in=w672) -> (error out=w671:errorcluster)  [unwired: 1 in, 2 out]
          }
          frame #4 {
            w677 = 1 ("length")
            n838 = local read "NAME"() -> (w678:string[])
            n839 = local read "VIRef"() -> (w683:refnum<vi>[])
            n840 = Delete From Array(array=w683, length=w677, index=w676) -> (array with subset deleted=w680:refnum<vi>[])  [unwired: 1 out]
            n841 = Delete From Array(array=w678, length=w677, index=w676) -> (array with subset deleted=w679:string[])  [unwired: 1 out]
            n842 = local read "ADRESS"() -> (w682:string[])
            n843 = local write "VIRef"(w680) -> ()
            n844 = local write "NAME"(w679) -> ()
            n845 = Delete From Array(array=w682, length=w677, index=w676) -> (array with subset deleted=w681:string[])  [unwired: 1 out]
            n846 = local write "ADRESS"(w681) -> ()
          }
          frame #5 {
            w685 = u8 0 ("Disabled")
            n847 = local write "DeleteChannel"(FALSE ("DeleteChannel")) -> ()
            n848 = property on="AddChannel" class="Bool (strict)"("Disabled"=w685) -> ()  [unwired: 2 in, 2 out]
            n849 = property on="CurrentModulationB" class="Bool (strict)"("Disabled"=w685) -> ()  [unwired: 2 in, 2 out]
            n850 = property on="DisconnectChannel" class="Bool (strict)"("Disabled"=w685) -> ()  [unwired: 2 in, 2 out]
            n851 = property on="ReadFromFile" class="Bool (strict)"("Disabled"=w685) -> ()  [unwired: 2 in, 2 out]
            n852 = property on="ConnectChannel" class="Bool (strict)"("Disabled"=w685) -> ()  [unwired: 2 in, 2 out]
            n853 = property on="Quit" class="Bool (strict)"("Disabled"=w685) -> ()  [unwired: 2 in, 2 out]
            n854 = property on="DeleteChannel" class="Bool (strict)"("Disabled"=w685) -> ()  [unwired: 2 in, 2 out]
            n855 = property on="WriteToFile" class="Bool (strict)"("Disabled"=w685) -> ()  [unwired: 2 in, 2 out]
            n856 = property on="Set Output ON All" class="Bool (strict)"("Disabled"=w685) -> ()  [unwired: 2 in, 2 out]
            n857 = property on="SetCurrentB" class="Bool (strict)"("Disabled"=w685) -> ()  [unwired: 2 in, 2 out]
            n858 = property on="ConnectAll" class="Bool (strict)"("Disabled"=w685) -> ()  [unwired: 2 in, 2 out]
            n859 = property on="SetOutputOnB" class="Bool (strict)"("Disabled"=w685) -> ()  [unwired: 2 in, 2 out]
            n860 = property on="SetVoltageB" class="Bool (strict)"("Disabled"=w685) -> ()  [unwired: 2 in, 2 out]
            n861 = property on="SetOutputOffB" class="Bool (strict)"("Disabled"=w685) -> ()  [unwired: 2 in, 2 out]
            n862 = property on="SetVoltageAll" class="Bool (strict)"("Disabled"=w685) -> ()  [unwired: 2 in, 2 out]
            n863 = property on="SetCurrentAll" class="Bool (strict)"("Disabled"=w685) -> ()  [unwired: 2 in, 2 out]
            n864 = property on="DisconnectAll" class="Bool (strict)"("Disabled"=w685) -> ()  [unwired: 2 in, 2 out]
          }
        }
      }
    }
    n865 = call <vilib>:"General Error Handler.vi"("type of dialog (OK msg:1)"=u8 0 ("Disabled"), "error in (no error)"=w120) -> ()  [unwired: 14 out]
  }
  n866 = while {
    stop <- FALSE stop-if-true
    n867 = property on="AddChannel" class="Bool (strict)"() -> ("Disabled"=w693:u8)  [unwired: 2 in, 2 out]
    n868 = local read "Quit"() -> (w691:bool)
    n869 = Not(x=w691) -> (.not. x?=w690:bool)
    n870 = Equal?(x=w693, y=u8 0) -> (x = y?=w689:bool)
    n871 = And(x=w690, y=w689) -> (x .and. y?=w688:bool)
    n872 = case shown="True" w688 {
      frame False {
      }
      frame True {
        w699 = string[] [] ("GlobalInAdress")
        n873 = local read "VIRef"() -> (w706:refnum<vi>[])
        n874 = Array Size(array=w706) -> (size(s)=w698:i32)
        n875 = for {
          N: w698 -> [_]
          tunnel: w706 -> [w775]
          shift-right: [w710] -> w697
          shift-left: w699 -> [w707]
          shift-right: [w709] -> w696
          shift-left: w699 -> [w708]
          shift-right: [w766] -> w694
          shift-left: w699 -> [w767]
          shift-right: [w755] -> w695
          shift-left: w699 -> [w762]
          shift-right: [w759] -> w702
          shift-left: w699 -> [w739]
          shift-right: [w753] -> w701
          shift-left: w699 -> [w754]
          i -> [w735]
          w752 = "" ("Control Name")
          n876 = Index Array(array=w775, index=w735) -> (element=w738:refnum<vi>)
          n877 = invoke class="VI" method="Ctrl Val.Get"(reference=w738, "Control Name"="SetVoltageStr") -> (error out=w747:errorcluster, "Get Control Value Variant"=w765:variant)  [unwired: 2 in, 2 out]
          n878 = invoke class="VI" method="Ctrl Val.Get"(reference=w738, "Control Name"="SetCurrentStr") -> (error out=w746:errorcluster, "Get Control Value Variant"=w764:variant)  [unwired: 2 in, 2 out]
          n879 = invoke class="VI" method="Ctrl Val.Get"(reference=w738, "Control Name"="Error") -> (error out=w733:errorcluster, "Get Control Value Variant"=w740:variant)  [unwired: 2 in, 2 out]
          n880 = invoke class="VI" method="Ctrl Val.Get"(reference=w738, "Control Name"="GetCurrent") -> (error out=w749:errorcluster, "Get Control Value Variant"=w772:variant)  [unwired: 2 in, 2 out]
          n881 = invoke class="VI" method="Ctrl Val.Get"(reference=w738, "Control Name"="GetVoltage") -> (error out=w748:errorcluster, "Get Control Value Variant"=w773:variant)  [unwired: 2 in, 2 out]
          n882 = invoke class="VI" method="Ctrl Val.Get"(reference=w738, "Control Name"="Output") -> (error out=w745:errorcluster, "Get Control Value Variant"=w756:variant)  [unwired: 2 in, 2 out]
          n883 = invoke class="VI" method="Ctrl Val.Get"(reference=w738, "Control Name"="Active") -> (error out=w744:errorcluster, "Get Control Value Variant"=w761:variant)  [unwired: 2 in, 2 out]
          n884 = Variant To Data(type=w752, Variant=w765) -> (data=w712:string)  [unwired: 1 in, 1 out]
          n885 = Variant To Data(type=w752, Variant=w764) -> (data=w717:string)  [unwired: 1 in, 1 out]
          n886 = Merge Errors(w733, w749, w748, w747) -> (w743:errorcluster)
          n887 = Merge Errors(w746, w745, w744) -> (w742:errorcluster)
          n888 = Variant To Data(type=w752, Variant=w772) -> (data=w769:string)  [unwired: 1 in, 1 out]
          n889 = Variant To Data(type=w752, Variant=w773) -> (data=w770:string)  [unwired: 1 in, 1 out]
          n890 = Variant To Data "Out"(type=w752, Variant=w756) -> (data=w741:string)  [unwired: 1 in, 1 out]
          n891 = String Length(string=w712) -> (length=w713:i32)
          n892 = String Length(string=w717) -> (length=w720:i32)
          n893 = Variant To Data(type=FALSE, Variant=w740) -> (data=w728:bool)  [unwired: 1 in, 1 out]
          n894 = disable-structure shown="Enabled" {
            disable-tunnel: [w786 w787] -> w729
            disable-tunnel: _ -> [w785 _]
            disable-tunnel: w728 -> [w784 w787]
            frame Disabled {
              n895 = Or(x=w784, y=w785) -> (x .or. y?=w786:bool)
            }
            frame Enabled {
            }
          }
          n896 = case shown="6, Default" w713 {
            tunnel: [4 ("milliseconds to wait") 5 ("milliseconds to wait")] -> w714
            tunnel: [0 ("milliseconds to wait") 0 ("milliseconds to wait")] -> w715
            frame 6, Default {
            }
            frame 7 {
            }
          }
          n897 = Variant To Data "Active"(type=FALSE, Variant=w761) -> (data=w727:bool)  [unwired: 1 in, 1 out]
          n898 = case shown="7" w720 {
            tunnel: [4 ("milliseconds to wait") 5 ("milliseconds to wait")] -> w719
            tunnel: [0 ("milliseconds to wait") 0 ("milliseconds to wait")] -> w718
            frame 6, Default {
            }
            frame 7 {
            }
          }
          n899 = Build Array (concatenate)(w707, w769) -> (w710:string[])
          n900 = Build Array (concatenate)(w708, w770) -> (w709:string[])
          n901 = case shown="True" w729 {
            tunnel: w738 -> [_ w838]
            tunnel: w735 -> [w820 w826]
            tunnel: [w819 w824] -> w730
            frame False {
              n902 = Bundle(w820, "milliseconds to wait"=8) -> (w821:cluster{i32, "milliseconds to wait":i32})  [unwired: 1 in]
              n903 = property on="error" class="MCListbox (strict)"("ActiveCell"=w821, "CellBG"=u32 16777225) -> (error out=w819:errorcluster)  [unwired: 2 in, 1 out]
            }
            frame True {
              w828 = "Connect" ("Control Name")
              n904 = invoke class="VI" method="Ctrl Val.Set"(reference=w838, "Control Name"=w828, "Value"=FALSE ("OK Button")) -> (reference out=w830:refnum<vi>, error out=w833:errorcluster)  [unwired: 2 in, 3 out]
              n905 = flat-sequence {
                tunnel: w833 -> [w843]
                tunnel: [w843] -> w831
                tunnel: w830 -> [w841]
                tunnel: [w841] -> w829
                tunnel: w828 -> [w840]
                tunnel: [w840] -> w827
                tunnel: w826 -> [w839]
                tunnel: [w839] -> w825
                frame #0 {
                  n906 = Wait (ms)(milliseconds to wait=u32 2000) -> ()  [unwired: 1 out]
                }
              }
              n907 = Bundle(w825, "milliseconds to wait"=8) -> (w835:cluster{i32, "milliseconds to wait":i32})  [unwired: 1 in]
              n908 = invoke class="VI" method="Ctrl Val.Set"(reference=w829, error in=w831, "Control Name"=w827, "Value"=TRUE ("OK Button")) -> (error out=w824:errorcluster)  [unwired: 1 in, 4 out]
              n909 = property on="error" class="MCListbox (strict)"("ActiveCell"=w835, "CellBG"=u32 16711680) -> ()  [unwired: 2 in, 2 out]
            }
          }
          n910 = case shown="\"1\"" w741 {
            tunnel: ["+" ("Control Name") "" ("Control Name") "-" ("Control Name")] -> w732
            tunnel: w735 -> [w788 w793 w798]
            frame "1" {
              n911 = Bundle(w788, "milliseconds to wait"=6) -> (w790:cluster{i32, "milliseconds to wait":i32})  [unwired: 1 in]
              n912 = property on="out" class="MCListbox (strict)"("ActiveCell"=w790, "CellBG"=u32 5895331) -> ()  [unwired: 2 in, 2 out]
            }
            frame Default {
              n913 = Bundle(w793, "milliseconds to wait"=6) -> (w795:cluster{i32, "milliseconds to wait":i32})  [unwired: 1 in]
              n914 = property on="out" class="MCListbox (strict)"("ActiveCell"=w795, "CellBG"=u32 16777225) -> ()  [unwired: 2 in, 2 out]
            }
            frame "0" {
              n915 = Bundle(w798, "milliseconds to wait"=6) -> (w800:cluster{i32, "milliseconds to wait":i32})  [unwired: 1 in]
              n916 = property on="out" class="MCListbox (strict)"("ActiveCell"=w800, "CellBG"=u32 13816530) -> ()  [unwired: 2 in, 2 out]
            }
          }
          n917 = String Subset(string=w712, offset (0)=w715, length (rest)=w714) -> (substring=w711:string)
          n918 = String Subset(string=w717, offset (0)=w718, length (rest)=w719) -> (substring=w716:string)
          n919 = case shown="False" w727 {
            tunnel: ["-" ("Control Name") "+" ("Control Name")] -> w760
            tunnel: w735 -> [w805 w814]
            tunnel: w732 -> [_ w813]
            tunnel: ["?" ("Control Name") w813] -> w731
            frame False {
              n920 = Bundle(w805, "milliseconds to wait"=7) -> (w811:cluster{i32, "milliseconds to wait":i32})  [unwired: 1 in]
              n921 = property on="active" class="MCListbox (strict)"("ActiveCell"=w811, "CellBG"=u32 14869218) -> (error out=w806:errorcluster)  [unwired: 2 in, 1 out]
              n922 = Bundle(w805, "milliseconds to wait"=6) -> (w804:cluster{i32, "milliseconds to wait":i32})  [unwired: 1 in]
              n923 = property on="out" class="MCListbox (strict)"(error in=w806, "ActiveCell"=w804, "CellBG"=u32 14869218) -> ()  [unwired: 1 in, 2 out]
            }
            frame True {
              n924 = Bundle(w814, "milliseconds to wait"=7) -> (w816:cluster{i32, "milliseconds to wait":i32})  [unwired: 1 in]
              n925 = property on="active" class="MCListbox (strict)"("ActiveCell"=w816, "CellBG"=u32 5895331) -> ()  [unwired: 2 in, 2 out]
            }
          }
          n926 = Merge Errors(w743, w742, w730) -> (w737:errorcluster)
          n927 = Search and Replace String(input string=w711, search string=",", replace string="." ("replace string (\"\")")) -> (result string=w724:string)  [unwired: 5 in, 3 out]
          n928 = Search and Replace String(input string=w716, search string=",", replace string="." ("replace string (\"\")")) -> (result string=w722:string)  [unwired: 5 in, 3 out]
          n929 = Build Array (concatenate)(w767, w724) -> (w766:string[])
          n930 = Build Array (concatenate)(w762, w722) -> (w755:string[])
          n931 = Build Array (concatenate)(w754, w731) -> (w753:string[])
          n932 = Build Array (concatenate)(w739, w760) -> (w759:string[])
          n933 = call <vilib>:"General Error Handler.vi"("type of dialog (OK msg:1)"=u32 0 ("milliseconds to wait"), "error in (no error)"=w737) -> ()  [unwired: 9 in, 5 out]
        }
        n934 = local read "ADRESS"() -> (w704:string[])
        n935 = local read "NAME"() -> (w703:string[])
        n936 = Build Array(w703, w704, w697, w696, w695, w694, w701, w702) -> (w705:string[][])
        n937 = Transpose 2D Array(2D array=w705) -> (transposed array=w700:string[][])
        n938 = property on="List of channels" class="MCListbox (strict)"("ItemNames"=w700) -> ()  [unwired: 2 in, 2 out]
      }
    }
  }
  n939 = property on="CurrentModulationB" class="Bool (strict)"(error in=w37, "Disabled"=w38) -> (error out=w36:errorcluster)  [unwired: 1 in, 1 out]
  n940 = property on="DisconnectAll" class="Bool (strict)"(error in=w30, "Disabled"=w38) -> (error out=w29:errorcluster)  [unwired: 1 in, 1 out]
  n941 = property on="DisconnectChannel" class="Bool (strict)"(error in=w36, "Disabled"=w38) -> (error out=w35:errorcluster)  [unwired: 1 in, 1 out]
  n942 = property on="WriteToFile" class="Bool (strict)"(error in=w29, "Disabled"=w38) -> (error out=w28:errorcluster)  [unwired: 1 in, 1 out]
  n943 = while {
    stop <- FALSE stop-if-true
    n944 = property on="List of channels" class="MCListbox (strict)"() -> ("ItemNames"=w850:string[][])  [unwired: 2 in, 2 out]
    n945 = Get Date/Time String(want seconds? (F)=TRUE) -> (date string=→"Дата":string, time string=→"Время":string)  [unwired: 2 in]
    n946 = Wait Until Next ms Multiple(millisecond multiple=u16 1000) -> ()  [unwired: 1 out]
    n947 = Empty Array?(array=w850) -> (empty?=w849:bool)
    n948 = case shown="False" w849 {
      tunnel: [T2."Enabled" ("Disabled") T2."Disabled and Grayed Out" ("Disabled")] -> w844
      frame False {
      }
      frame True {
      }
    }
    n949 = property on="Common curr. inc" class="Bool (strict)"("DisabledEnum"=w844) -> ()  [unwired: 2 in, 2 out]
    n950 = property on="Common curr. dec" class="Bool (strict)"("DisabledEnum"=w844) -> ()  [unwired: 2 in, 2 out]
    n951 = property on="Set Output ON All" class="Bool (strict)"("DisabledEnum"=w844) -> ()  [unwired: 2 in, 2 out]
    n952 = property on="Common volt. inc" class="Bool (strict)"("DisabledEnum"=w844) -> ()  [unwired: 2 in, 2 out]
    n953 = property on="DisconnectAll" class="Bool (strict)"("DisabledEnum"=w844) -> ()  [unwired: 2 in, 2 out]
    n954 = property on="SetVoltageB" class="Bool (strict)"("DisabledEnum"=w844) -> ()  [unwired: 2 in, 2 out]
    n955 = property on="ConnectChannel" class="Bool (strict)"("DisabledEnum"=w844) -> ()  [unwired: 2 in, 2 out]
    n956 = property on="SetOutputOnB" class="Bool (strict)"("DisabledEnum"=w844) -> ()  [unwired: 2 in, 2 out]
    n957 = property on="DisconnectChannel" class="Bool (strict)"("DisabledEnum"=w844) -> ()  [unwired: 2 in, 2 out]
    n958 = property on="SetOutputOffB" class="Bool (strict)"("DisabledEnum"=w844) -> ()  [unwired: 2 in, 2 out]
    n959 = property on="ConnectAll" class="Bool (strict)"("DisabledEnum"=w844) -> ()  [unwired: 2 in, 2 out]
    n960 = property on="SetCurrentB" class="Bool (strict)"("DisabledEnum"=w844) -> ()  [unwired: 2 in, 2 out]
  }
  n961 = property on="SetCurrentB" class="Bool (strict)"(error in=w28, "Disabled"=w38) -> (error out=w27:errorcluster)  [unwired: 1 in, 1 out]
  n962 = property on="ConnectAll" class="Bool (strict)"(error in=w35, "Disabled"=w38) -> (error out=w34:errorcluster)  [unwired: 1 in, 1 out]
  n963 = property on="SelectedBuvSetVolB" class="Bool"("DisabledEnum"=T2."Enabled" ("Disabled")) -> ()  [unwired: 2 in, 2 out]
  n964 = property on="Quit" class="Bool (strict)"(error in=w27, "Disabled"=w38) -> (error out=w26:errorcluster)  [unwired: 1 in, 1 out]
  n965 = property on="ReadFromFile" class="Bool (strict)"(error in=w34, "Disabled"=w38) -> (error out=w33:errorcluster)  [unwired: 1 in, 1 out]
  n966 = call <vilib>:"Application Directory.vi"() -> ("Application Directory"=w18:path)
  n967 = Build Path(base path=w18, name or relative path="BuvConfig.dat") -> (appended path=w15:path)
  n968 = property on="SetOutputOnB" class="Bool (strict)"(error in=w26, "Disabled"=w38) -> (error out=w25:errorcluster)  [unwired: 1 in, 1 out]
  n969 = property on="ConnectChannel" class="Bool (strict)"(error in=w33, "Disabled"=w38) -> (error out=w32:errorcluster)  [unwired: 1 in, 1 out]
  n970 = Open/Create/Replace File(file path (use dialog)=w15, operation (0:open)=T1."open") -> (refnum out=w13:refnum<file>, error out=w14:errorcluster)  [unwired: 4 in, 1 out]
  n971 = Read from Text File(file (use dialog)=w13, error in=w14) -> (text=w10:string, error out=w5:errorcluster)  [unwired: 2 in, 2 out]
  n972 = property on="SetVoltageB" class="Bool (strict)"(error in=w25, "Disabled"=w38) -> (error out=w24:errorcluster)  [unwired: 1 in, 1 out]
  n973 = Match Pattern(string=w10, regular expression="Z" ("string")) -> (before substring=w9:string, after substring=w6:string)  [unwired: 1 in, 2 out]
  n974 = property on="SetOutputOffB" class="Bool (strict)"(error in=w24, "Disabled"=w38) -> ()  [unwired: 1 in, 2 out]
  n975 = property on="DeleteChannel" class="Bool (strict)"(error in=w32, "Disabled"=w38) -> (error out=w31:errorcluster)  [unwired: 1 in, 1 out]
  n976 = Scan From String(input string=w6, error in=w5) -> (error out=w2:errorcluster, output 1=w7:dbl)  [unwired: 3 in, 2 out]
  n977 = Scan From String(input string=w9, error in=w2, default 1=u16 0 ("default value 1")) -> (error out=w4:errorcluster, output 1=w12:u16)  [unwired: 2 in, 2 out]
  n978 = local write "SelectedBuvOutVolt"(w7) -> ()
  n979 = case shown="No Error" w4 {
    selector: w4 -> [w854 w856]
    tunnel: [TRUE ("LoadPhase") FALSE ("LoadPhase")] -> w3
    tunnel: [w854 w856] -> w1
    frame No Error {
    }
    frame Error {
    }
  }
  "LoadPhase" <- w3
  n980 = local write "SelectedBuvPhase"(w12) -> ()
  n981 = property on="SetVoltageAll" class="Bool (strict)"(error in=w31, "Disabled"=w38) -> ()  [unwired: 1 in, 2 out]
  n982 = while {
    tunnel: w1 -> [w860]
    stop <- FALSE stop-if-true
    n983 = flat-sequence {
      tunnel: [w873] -> w868
      tunnel: [w872] -> w867
      tunnel: w860 -> [w871]
      tunnel: w868 -> [w880]
      tunnel: w867 -> [w879]
      tunnel: [w878] -> w866
      tunnel: [w877] -> w865
      tunnel: w866 -> [w939]
      tunnel: [w938] -> w864
      tunnel: w865 -> [w937]
      tunnel: [w936] -> w863
      tunnel: w864 -> [w1008]
      tunnel: w863 -> [w1007]
      tunnel: [w988] -> w862
      tunnel: [w986] -> w861
      tunnel: w862 -> [w1065]
      tunnel: w861 -> [w1062]
      frame #0 {
        n984 = TCP Open Connection(address="172.16.21.81", remote port or service name=u16 4001, timeout ms (60000)=1000, error in (no error)=w871) -> (connection ID=w872:refnum<k5>, error out=w873:errorcluster)  [unwired: 1 in]
        "Buv con ID" <- w872
      }
      frame #1 {
        n985 = case shown="No Error" w880 {
          selector: w880 -> [w882 w935]
          tunnel: w879 -> [w884 w934]
          tunnel: [w883 w935] -> w878
          tunnel: [w881 w934] -> w877
          frame No Error {
            n986 = local read "LoadVolt"() -> (w886:bool)
            n987 = Or(x="SelectedBuvSetVolB", y=w886) -> (x .or. y?=w885:bool)
            n988 = case shown="True" w885 {
              tunnel: [w889 w893] -> w881
              tunnel: [w888 w892] -> w883
              tunnel: w884 -> [w889 w900]
              tunnel: w882 -> [w888 _]
              frame False {
              }
              frame True {
                # "Пустое считывание,\nнеобх. после команды"
                # "Установка опорного напряжения"
                n989 = local read "SelectedBuvPhase"() -> (w918:u16)
                n990 = Divide(x="SelectedBuvOutVolt", y=0.125) -> (x/y=w921:dbl)
                n991 = To Unsigned Word Integer(number=w921) -> (unsigned 16bit integer=w928:u16)
                n992 = Format Into String(format string="%d", w918) -> (resulting string=w919:string, error out=w902:errorcluster)  [unwired: 2 in]
                n993 = Format Into String(format string="%.1f", "SelectedBuvOutVolt") -> (resulting string=w913:string, error out=w903:errorcluster)  [unwired: 2 in]
                n994 = Format Into String(format string="%04d", w928) -> (resulting string=w925:string, error out=w904:errorcluster)  [unwired: 2 in]
                n995 = local write "LoadVolt"(FALSE ("LoadPhase")) -> ()
                n996 = Concatenate Strings(w919, "Z" ("string"), w913) -> (w912:string)
                n997 = Merge Errors(w902, w903, w904) -> (w901:errorcluster)
                n998 = Concatenate Strings("r" ("data in"), w925) -> (w926:string)
                n999 = TCP Write(connection ID=w900, data in=w926, 9:2000 ("timeout ms (25000)")) -> (connection ID out=w923:refnum<k5>, error out=w922:errorcluster)  [unwired: 1 in, 1 out]
                n1000 = call <vilib>:"Application Directory.vi"() -> ("Application Directory"=w910:path)
                n1001 = flat-sequence {
                  tunnel: [w933] -> w891
                  tunnel: w923 -> [w933]
                  tunnel: [w932] -> w890
                  tunnel: w922 -> [w932]
                  frame #0 {
                    n1002 = Wait (ms)(milliseconds to wait=u32 100) -> ()  [unwired: 1 out]
                  }
                }
                n1003 = Build Path(base path=w910, name or relative path="BuvConfig.dat") -> (appended path=w909:path)
                n1004 = Open/Create/Replace File(file path (use dialog)=w909, error in=w901) -> (refnum out=w916:refnum<file>, error out=w915:errorcluster)  [unwired: 4 in, 1 out]
                n1005 = Write to Text File(file (use dialog)=w916, text=w912, error in=w915) -> (error out=w906:errorcluster)  [unwired: 1 in, 2 out]
                n1006 = TCP Write(connection ID=w891, data in="u", error in (no error)=w890) -> (connection ID out=w898:refnum<k5>, error out=w894:errorcluster)  [unwired: 1 in, 1 out]
                n1007 = call <vilib>:"General Error Handler.vi"("type of dialog (OK msg:1)"=u32 0 ("milliseconds to wait"), "error in (no error)"=w906) -> ()  [unwired: 9 in, 5 out]
                n1008 = TCP Read(connection ID=w898, bytes to read=11, error in (no error)=w894, 7:T5."Standard" ("mode (standard)"), 9:2000 ("timeout ms (25000)")) -> (connection ID out=w893:refnum<k5>, error out=w892:errorcluster)  [unwired: 1 out]
              }
            }
          }
          frame Error {
          }
        }
      }
      frame #2 {
        n1009 = case shown="No Error" w939 {
          selector: w939 -> [w942 w985]
          tunnel: [w943 w985] -> w938
          tunnel: w937 -> [w941 w984]
          tunnel: [w940 w984] -> w936
          frame No Error {
            n1010 = local read "LoadPhase"() -> (w945:bool)
            n1011 = Or(x="BuvPhaseSetB", y=w945) -> (x .or. y?=w944:bool)
            n1012 = case shown="True" w944 {
              tunnel: [w947 w950] -> w940
              tunnel: [w948 w949] -> w943
              tunnel: w942 -> [w948 _]
              tunnel: w941 -> [w947 w959]
              frame False {
              }
              frame True {
                # "Пустое считывание,\nнеобх. после команды"
                # "Установка фазы"
                n1013 = local write "LoadPhase"(FALSE ("LoadPhase")) -> ()
                n1014 = Format Into String(format string="%04d", "SelectedBuvPhase") -> (resulting string=w972:string)  [unwired: 2 in, 1 out]
                n1015 = Concatenate Strings("p" ("data in"), w972) -> (w978:string)
                n1016 = local read "SelectedBuvOutVolt"() -> (w971:dbl)
                n1017 = TCP Write(connection ID=w959, data in=w978, 9:2000 ("timeout ms (25000)")) -> (connection ID out=w975:refnum<k5>)  [unwired: 1 in, 2 out]
                n1018 = call <vilib>:"Application Directory.vi"() -> ("Application Directory"=w966:path)
                n1019 = Format Into String(format string="%.1f", w971) -> (resulting string=w969:string)  [unwired: 2 in, 1 out]
                n1020 = Build Path(base path=w966, name or relative path="BuvConfig.dat") -> (appended path=w965:path)
                n1021 = Open/Create/Replace File(file path (use dialog)=w965, operation (0:open)=T1."replace or create") -> (refnum out=w974:refnum<file>, error out=w973:errorcluster)  [unwired: 4 in, 1 out]
                n1022 = Concatenate Strings(w972, "Z" ("string"), w969) -> (w968:string)
                n1023 = Write to Text File(file (use dialog)=w974, text=w968, error in=w973) -> (error out=w962:errorcluster)  [unwired: 1 in, 2 out]
                n1024 = flat-sequence {
                  tunnel: [w983] -> w952
                  tunnel: w975 -> [w983]
                  tunnel: [w982] -> w951
                  tunnel: w962 -> [w982]
                  frame #0 {
                    n1025 = Wait (ms)(milliseconds to wait=u32 100) -> ()  [unwired: 1 out]
                    "LoadVolt" <- TRUE ("LoadVolt")
                  }
                }
                n1026 = TCP Write(connection ID=w952, data in="u", error in (no error)=w951) -> (connection ID out=w954:refnum<k5>, error out=w958:errorcluster)  [unwired: 1 in, 1 out]
                n1027 = TCP Read(connection ID=w954, bytes to read=11, error in (no error)=w958, 7:T5."Standard" ("mode (standard)"), 9:2000 ("timeout ms (25000)")) -> (connection ID out=w950:refnum<k5>, error out=w949:errorcluster)  [unwired: 1 out]
              }
            }
          }
          frame Error {
          }
        }
      }
      frame #3 {
        w987 = string[] [] ("GlobalInAdress")
        n1028 = case shown="No Error" w1008 {
          selector: w1008 -> [w1029 w1060]
          tunnel: w1007 -> [w1035 w1059]
          tunnel: [w1033 "*"] -> w995
          tunnel: [w1032 w1060] -> w989
          tunnel: [w1031 w1059] -> w988
          frame No Error {
            n1029 = TCP Write(connection ID=w1035, data in="u", error in (no error)=w1029) -> (connection ID out=w1037:refnum<k5>, error out=w1041:errorcluster)  [unwired: 1 in, 1 out]
            n1030 = TCP Read(connection ID=w1037, bytes to read=11, error in (no error)=w1041, 7:T5."CRLF" ("mode (standard)"), 9:2000 ("timeout ms (25000)")) -> (connection ID out=w1030:refnum<k5>, data out=w1034:string, error out=w1042:errorcluster)
            n1031 = case shown="No Error" w1042 {
              selector: w1042 -> [_ w1057]
              tunnel: [w1052 "-"] -> w1033
              tunnel: w1034 -> [w1045 _]
              tunnel: [w1044 w1057] -> w1032
              tunnel: [w1043 w1056] -> w1031
              tunnel: w1030 -> [w1043 w1056]
              frame No Error {
                n1032 = Match Pattern(string=w1045, regular expression="=") -> (after substring=w1046:string)  [unwired: 1 in, 3 out]
                n1033 = Scan From String(format string="%f", input string=w1046, default 1=0.0 ("default value 1")) -> (error out=w1048:errorcluster, output 1=w1051:dbl)  [unwired: 2 in, 2 out]
                n1034 = Multiply(x=w1051, y=0.125) -> (x*y=w1050:dbl)
                n1035 = Format Into String(format string="%.1f", error in=w1048, w1050) -> (resulting string=w1052:string, error out=w1044:errorcluster)  [unwired: 1 in]
              }
              frame Error {
              }
            }
          }
          frame Error {
          }
        }
        n1036 = case shown="No Error" w989 {
          selector: w989 -> [w1013 w1023]
          tunnel: ["-" ("Control Name") "+" ("Control Name")] -> w992
          tunnel: [w1013 w1023] -> w986
          frame Error {
            n1037 = Bundle("milliseconds to wait"=0, "milliseconds to wait"=4) -> (w1011:T6)  [unwired: 1 in]
            n1038 = property on="Buv Table" class="MCListbox (strict)"("ActiveCell"=w1011, "CellBG"=u32 16725248) -> ()  [unwired: 2 in, 2 out]
            n1039 = Bundle("milliseconds to wait"=0, "milliseconds to wait"=3) -> (w1015:T6)  [unwired: 1 in]
            n1040 = property on="Buv Table" class="MCListbox (strict)"("ActiveCell"=w1015, "CellBG"=u32 13816530) -> ()  [unwired: 2 in, 2 out]
          }
          frame No Error {
            n1041 = Bundle("milliseconds to wait"=0, "milliseconds to wait"=4) -> (w1022:T6)  [unwired: 1 in]
            n1042 = property on="Buv Table" class="MCListbox (strict)"("ActiveCell"=w1022, "CellBG"=u32 16448250) -> ()  [unwired: 2 in, 2 out]
            n1043 = Bundle("milliseconds to wait"=0, "milliseconds to wait"=3) -> (w1024:T6)  [unwired: 1 in]
            n1044 = property on="Buv Table" class="MCListbox (strict)"("ActiveCell"=w1024, "CellBG"=u32 5895331) -> ()  [unwired: 2 in, 2 out]
          }
        }
        n1045 = property on="SelectedBuvOutVolt" class="DigNum (strict)"() -> ("Value"=w1002:dbl)  [unwired: 2 in, 2 out]
        n1046 = Format Into String(format string="%.1f", w1002) -> (resulting string=w1000:string)  [unwired: 2 in, 1 out]
        n1047 = Build Array (concatenate)(w992, string[] [] ("GlobalInAdress")) -> (w990:string[])
        n1048 = Build Array (concatenate)(w1000, string[] [] ("GlobalInAdress")) -> (w999:string[])
        n1049 = Build Array (concatenate)(w995, string[] [] ("GlobalInAdress")) -> (w994:string[])
        n1050 = Build Array (concatenate)("1" ("address"), string[] [] ("GlobalInAdress")) -> (w1005:string[])
        n1051 = Build Array(w987, w987) -> (w997:string[][])
        n1052 = Build Array (concatenate)(w1005, w994, w999, w990, w997) -> (w1003:string[][])
        n1053 = Transpose 2D Array(2D array=w1003) -> (transposed array=w1004:string[][])
        n1054 = property on="Buv Table" class="MCListbox (strict)"("ItemNames"=w1004) -> ()  [unwired: 2 in, 2 out]
      }
      frame #4 {
        n1055 = case shown="Error" w1062 {
          frame No Error {
          }
          frame Error {
            w1066 = TRUE ("LoadPhase")
            n1056 = local write "LoadPhase"(w1066) -> ()
            n1057 = local write "LoadVolt"(w1066) -> ()
          }
        }
        n1058 = TCP Close Connection(connection ID=w1065) -> (error out=w1064:errorcluster)  [unwired: 2 in, 1 out]
        n1059 = call <vilib>:"General Error Handler.vi"("type of dialog (OK msg:1)"=0 ("milliseconds to wait"), "error in (no error)"=w1064) -> ()  [unwired: 9 in, 5 out]
      }
    }
    n1060 = Wait Until Next ms Multiple(millisecond multiple=u32 70) -> ()  [unwired: 1 out]
    n1061 = Not(x="SetPhaseEn") -> (.not. x?=w858:bool)
    n1062 = property on="BuvPhaseSetB" class="Bool"("Visible"=w858) -> ()  [unwired: 2 in, 2 out]
    n1063 = property on="SelectedBuvPhase" class="DigNum (strict)"("Visible"=w858) -> ()  [unwired: 2 in, 2 out]
  }
  "VIRef" <- refnum<vi>[] []
  "ADRESS" <- string[] [] ("GlobalInAdress")
  "NAME" <- string[] [] ("GlobalInAdress")
  "CURRENTSET" <- dbl[] [] ("GlobalInAdress")
